vi "Laser manager 1.0BETA_withMotor.vi"() -> ()   [LabVIEW 2014]
uses:
  <vilib>/userdefined/High Color/IMAQdx.ctl
  Typedef/Consumer loop - States.ctl
  Typedef/UI data.ctl
  <vilib>/MakerHub/LINX/Public/Peripherals/Digital/Digital Write 1 Chan.vi
  <vilib>/MakerHub/LINX/Public/Peripherals/Digital/Digital Write N Chans.vi
  <vilib>/MakerHub/LINX/Private/Local IO/LinxDigitalWrite.vi
  <vilib>/MakerHub/LINX/Public/Utilities/Check Channel.vi
  <vilib>/MakerHub/LINX/Public/Utilities/Open Serial.vi
  <vilib>/MakerHub/LINX/Private/Utilties/Generate Error.vi
  <vilib>/vision/driver/NI_Vision_Acquisition_Software.lvlib
  <vilib>/MakerHub/LINX/LMH-LINX.lvlib
panel:
  in  "Move":bool
  in  "Absolute Y":dbl caption="Absolute Y [mm]"
  in  "Absolute X":dbl caption="Absolute X [mm]"
  in  "Delta Y":dbl caption="Delta Y [mm]"
  in  "Delta X":dbl caption="Delta X [mm]"
  in  "Move type":enum32{"Step mode", "\"Go to\" mode"}(radio)=enum."\"Go to\" mode"
  in  "Right":bool
  in  "Left":bool
  in  "Up":bool
  in  "Down":bool
  in  "Exit":bool
  out "Image":T1(plugin-control)
  in  "Tab Control":enum32{"Standard operations", "Refill", "Tools"}(tab)
  in  "Main - Open calib":bool
  in  "Go to calib":bool
  in  "Save calib":bool
  in  "Thyratron Bias [kV]":dbl=20.0
  in  "Test Laser":bool
  in  "Frequency [Hz]":u16=1 min=1 max=50 step=1
  in  "Beam Y":dbl=63.0 caption="Y" min=0.1 step=1.0 format="%#_gmm"
  in  "Beam X":dbl=1.0 caption="X" min=0.1 step=1.0 format="%#_gmm"
  in  "How to choose":bool
  in  "Load Pt2":bool
  out "X2":dbl format="%.2fmm"
  out "Y2":dbl format="%.2fmm"
  in  "Load Pt1":bool
  out "X1":dbl format="%.2fmm"
  out "Y1":dbl format="%.2fmm"
  in  "Abort":bool
  in  "Beam Overlap":dbl caption="Lateral Overlap [mm]" min=0.0 max=62.0 step=1.0
  in  "Shots/point":dbl=1.0 min=1.0 max=1000.0 step=1.0
  in  "Xspeed":dbl=1.0 caption="X speed [mm/s]" min=0.01 max=100.0 format="%#_3g"
  in  "Irradiate":bool
  out "Pressure":string caption="Pressure [mbar]"
  in  "Refill":bool
  in  "Purge Inert":bool
  in  "Purge Buffer":bool
  in  "Purge Rare":bool
  in  "Purge Halogen":bool
  in  "Set Gas Pressures [mbar]":T2={"Halogen"=80, "Rare"=60, "Buffer "=3160, "Inert"=0}
  out "Interface status":bool
  in  "Motor Enable":bool
  in  "Open GPIB interface":bool
  in  "Enable motors":bool
  in  "Find Origin":bool
  in  "Reset ESP":bool
  in  "Tools - Open Calib":bool
  in  "Open Attenuator":bool
  # "Free mode"
  # "LASER MANAGER 1.1 BETA"
  # "written by frax84"
  # "Energy Calibration"
  # "Laser Parameters"
  # "Beam parameters"
  # "Beam size"
  # "Motor path settings"
  # "Irradiation main controls"
  # "Purge Options"
  # "CAUTION\nEach purge operation \nlasts 5 seconds!"
  # "Reading is performed\nevery 5 seconds"
  # "Peripherals comunication"
  # "Gas mixing motor control"
  # "Motor Utilities"
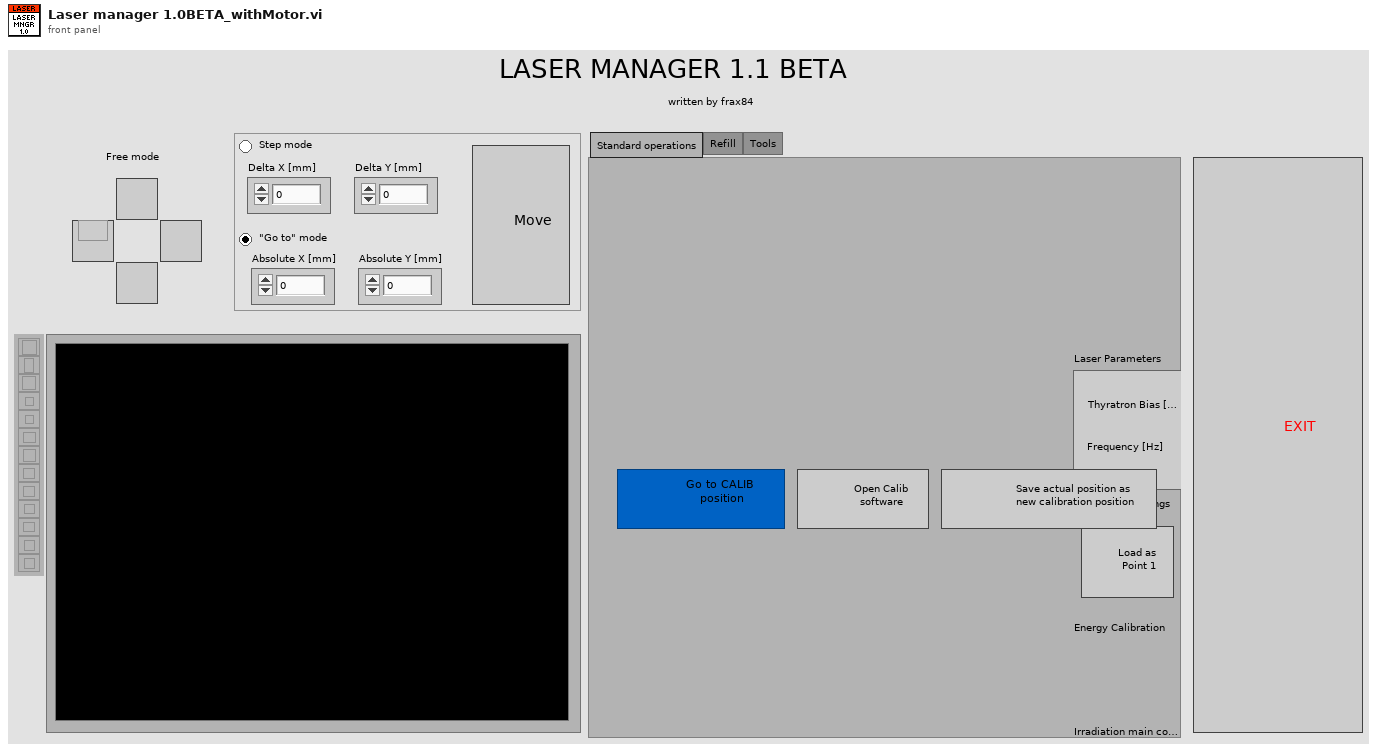
[diagram p1: front panel]
types:
  T1 = typedef "IMAQ Image.ctl" = refnum<image>
  T2 = cluster{"Halogen":u16, "Rare":u16, "Buffer ":u16, "Inert":u16}
  T3 = typedef "UI data.ctl" = cluster{"GPIB Addresses":cluster{"GPIB Motor":i16, "GPIB Laser":string}, "Beam size":cluster{"BeamX":dbl, "BeamY":dbl, "Beam Overlap":dbl}, "Motor speed":cluster{"Xspeed":dbl, " Yspeed":dbl}, "Laser parameters":cluster{"Thyratron Bias":dbl, "Frequency":u16, "Shots/Point":dbl}, "Irradiation points":cluster{"X1":dbl, "Y1":dbl, "X2":dbl, "Y2":dbl}, "Calibration Point":cluster{"Xcalib":dbl, "Ycalib":dbl}}
  T4 = typedef "Consumer loop - States.ctl" = enum16{"Idle", "Read Pressure", "Move up", "Move down", "Move left", "Move right", "Move to", "Move Delta", "Stop Motion", "Go to calib", "Check if move done", "Disable buttons", "Enable buttons", "Irradiation - Stop", "Irradiation - Check points", "Irradiation - Disable buttons", "Irradiation - Init position", "Irradiation - Check if done", "Irradiation - Sweep X", "Irradiation - Check X", "Irradiation - Check Y", "Irradiation - Sweep Y", "Irradiation - Enable buttons"}
  T5 = typedef "Image Type" = u32
  T6 = typedef "IMAQdx.ctl" = refnum<k21>
  T7 = enum8{"Enabled", "Disabled", "Disabled and Grayed Out"}
  T8 = typedef "LMH-LINX.lvlib/LINX Ref.ctl" = cluster{"IO":T9, "Interface":T10, "LINX Device Config":T11}
  T9 = typedef "LMH-LINX.lvlib/Platform.ctl" = enum16{"Remote", "Local"}
  T10 = typedef "LMH-LINX.lvlib/Interface.ctl" = enum16{"Serial", "TCP"}
  T11 = typedef "LMH-LINX.lvlib/Device.lvlib/LINX Device Config.ctl" = cluster{"Interface":T10, "COM Port":refnum<visa-resource-name>, "TCP Configuration":T12, "Device Family":u8, "Device ID":u8, "Device Name":string, "TCP Ref":refnum<k5>, "Channels":T13}
  T12 = typedef "LMH-LINX.lvlib/Device.lvlib/TCP Config.ctl" = cluster{"IP Address":string, "Port":u16}
  T13 = typedef "LMH-LINX.lvlib/Channels.ctl" = cluster{"DI":u8[], "DO":u8[], "AI":u8[], "AO":u8[], "PWM":u8[], "QE":u8[], "UART":u8[], "I2C 2":u8[], "SPI":u8[], "CAN":u8[], "Servo":u8[], "AI Ref (V)":dbl, "AI Resolution (Bits)":u8, "AO Ref (V)":dbl, "AO Resolution (Bits)":u8}
  T14 = cluster{"Global Rectangle":i32[], "Contours":cluster{"Contour Type":u32, "ROI Type":u32, "Points":i32[]}[]}
  T15 = cluster{"Global Rectangle[0]":i32, "Global Rectangle[1]":i32, "Global Rectangle[2]":i32, "Global Rectangle[3]":i32}
  T16 = cluster{"Consumer loop - States":T4, "Variant":variant}
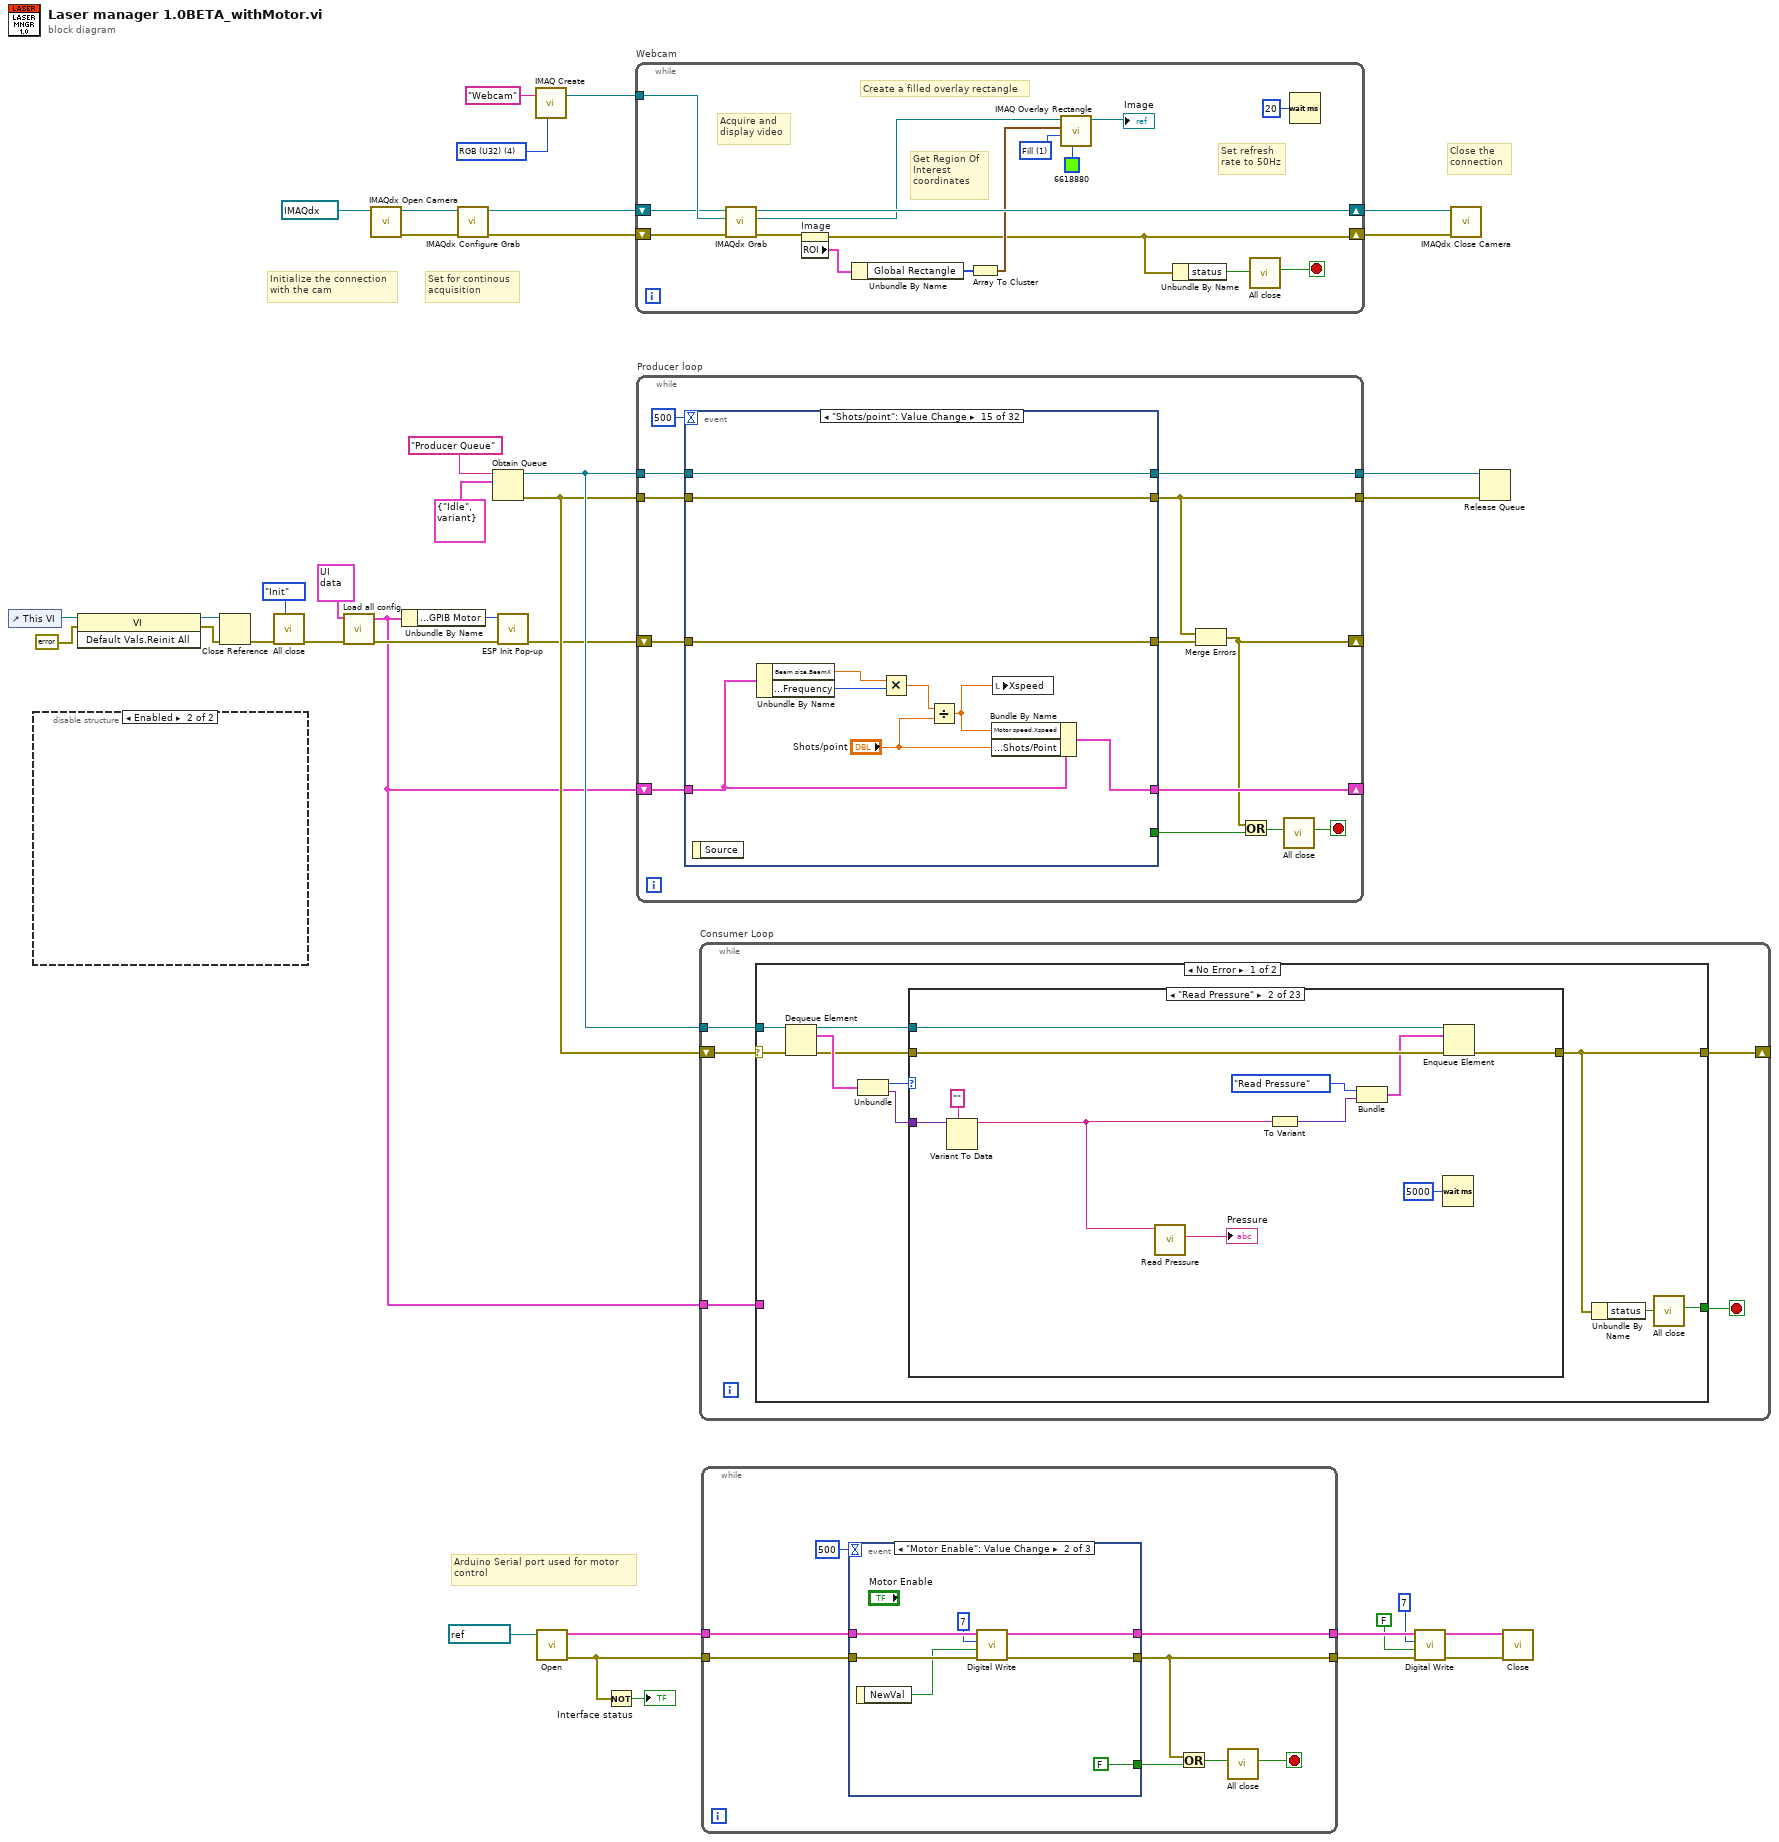
[diagram p0: block diagram]
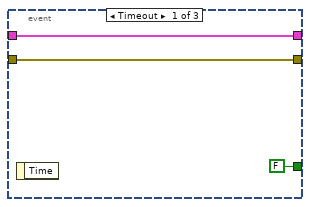
[diagram p2: hidden frame]
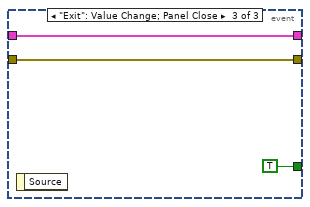
[diagram p3: hidden frame]
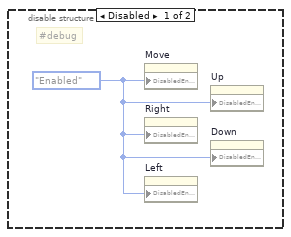
[diagram p4: hidden frame]
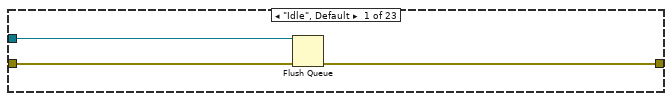
[diagram p5: hidden frame]
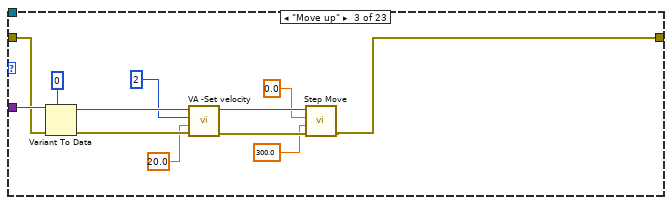
[diagram p6: hidden frame]
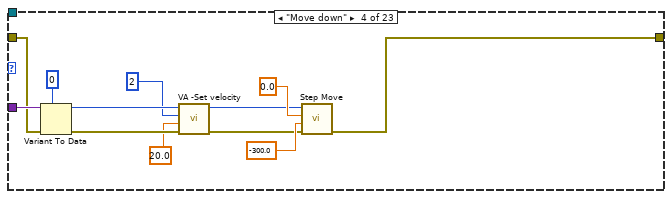
[diagram p7: hidden frame]
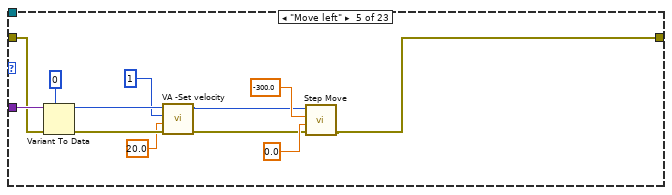
[diagram p8: hidden frame]
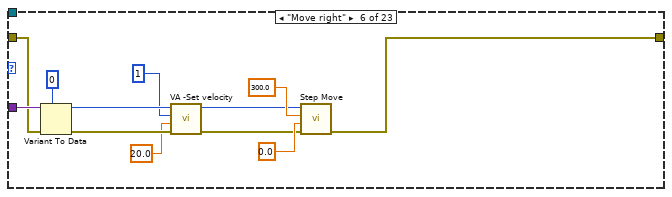
[diagram p9: hidden frame]
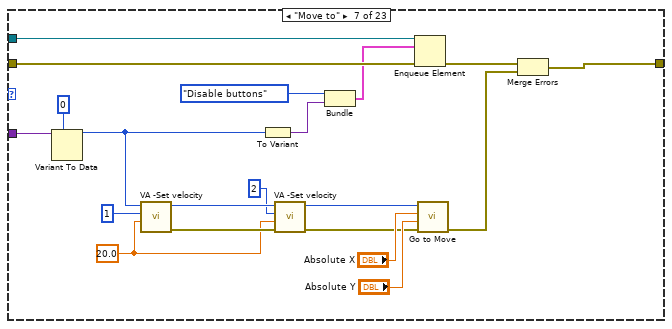
[diagram p10: hidden frame]
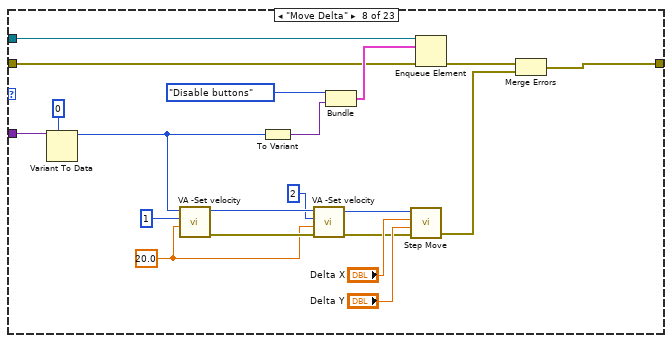
[diagram p11: hidden frame]
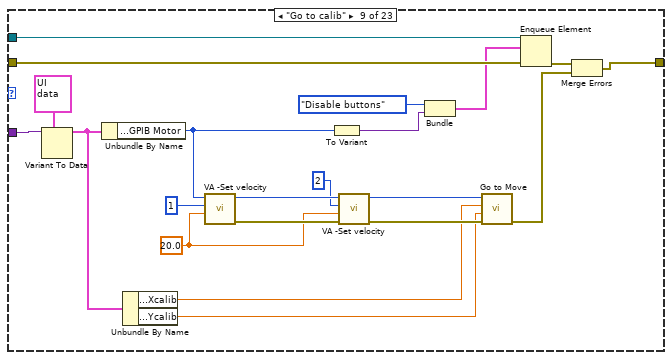
[diagram p12: hidden frame]
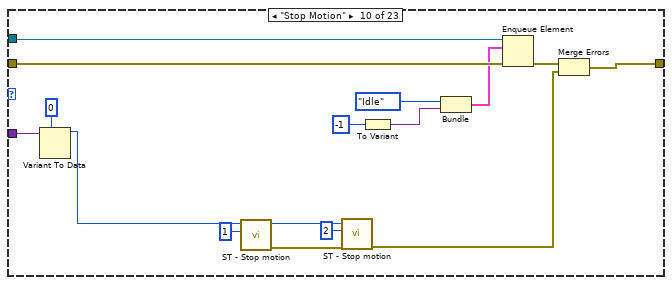
[diagram p13: hidden frame]
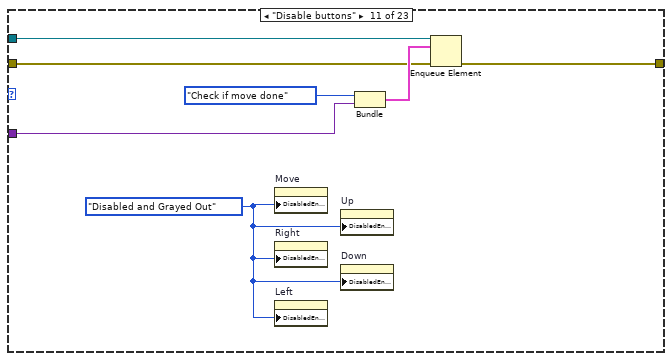
[diagram p14: hidden frame]
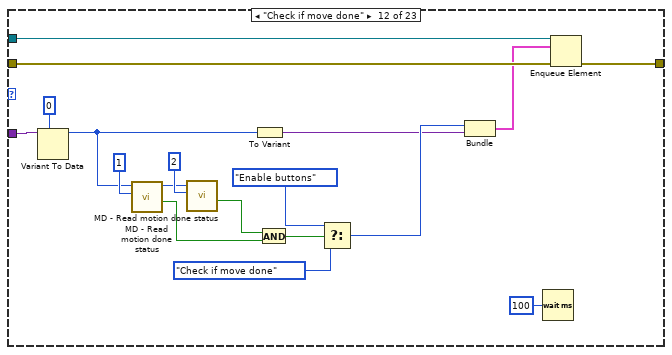
[diagram p15: hidden frame]
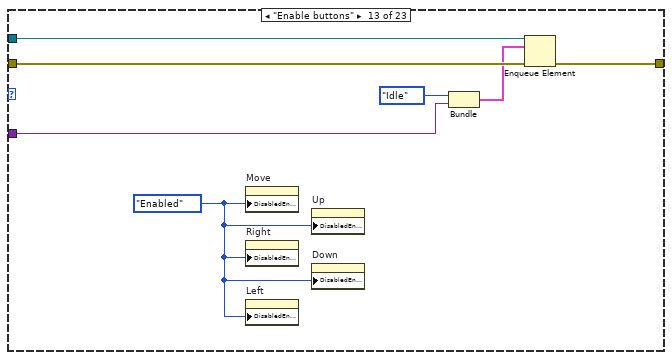
[diagram p16: hidden frame]
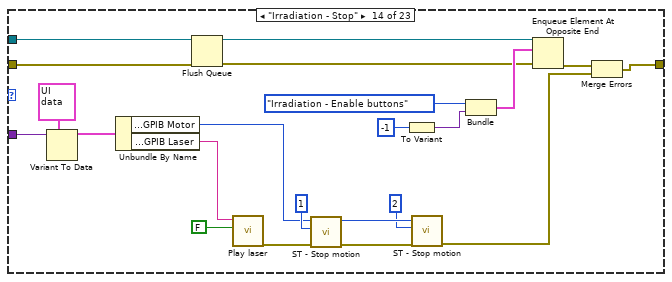
[diagram p17: hidden frame]
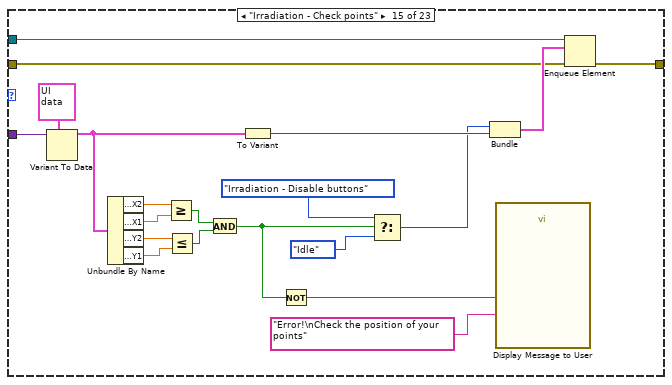
[diagram p18: hidden frame]
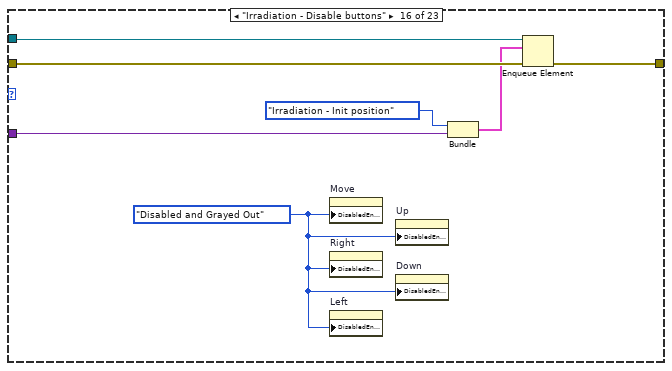
[diagram p19: hidden frame]
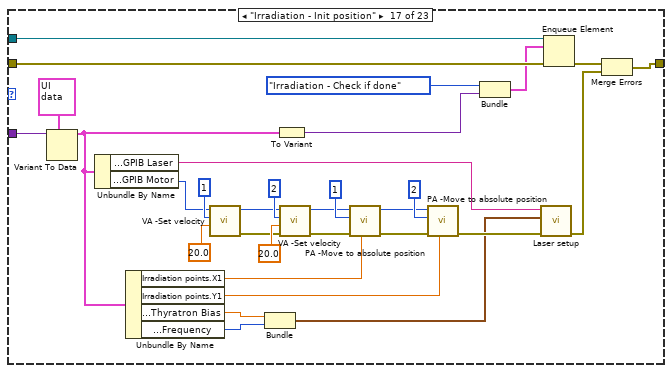
[diagram p20: hidden frame]
diagram:
  w32 = T5 4 items=["Grayscale (U8)", "Grayscale (I16)", "Grayscale (SGL)", "Complex (CSG)", "RGB (U32)", "HSL (U32)", "RGB (U64)", "Grayscale (U16)"] ("Image Type")
  # "Arduino Serial port used for motor\ncontrol"
  # "Close the \nconnection"
  # "Set for continous\nacquisition"
  # "Initialize the connection\nwith the cam"
  n1 = control-ref of="This VI"() -> (w15:refnum<vi>)
  n2 = disable-structure shown="Enabled" {
    frame Disabled {
      w39 = T7."Enabled" ("Disabled")
      # "#debug"
      n3 = property on="Move" class="Bool"("DisabledEnum"=w39) -> ()  [unwired: 2 in, 2 out]
      n4 = property on="Right" class="Bool (strict)"("DisabledEnum"=w39) -> ()  [unwired: 2 in, 2 out]
      n5 = property on="Left" class="Bool (strict)"("DisabledEnum"=w39) -> ()  [unwired: 2 in, 2 out]
      n6 = property on="Up" class="Bool (strict)"("DisabledEnum"=w39) -> ()  [unwired: 2 in, 2 out]
      n7 = property on="Down" class="Bool (strict)"("DisabledEnum"=w39) -> ()  [unwired: 2 in, 2 out]
    }
    frame Enabled {
    }
  }
  n8 = invoke class="VI" method="Default Vals.Reinit All"(reference=w15, error in=errorcluster {"status"=FALSE, "code"=0, "source"=""} ("Error In")) -> (reference out=w13:refnum<vi>, error out=w14:errorcluster)  [unwired: 1 in, 1 out]
  n9 = Close Reference(reference=w13, error in (no error)=w14) -> (error out=w12:errorcluster)
  n10 = call "All close.vi"("Operation (Check)"=enum16{"Init", "Check"}."Init" ("Operation"), "Error In"=w12) -> ("Error Out"=w18:errorcluster)  [unwired: 8 in, 1 out]
  n11 = call "Load all config.vi"("Error In"=w18, "UI data in"=T3 {"GPIB Addresses"={"GPIB Motor"=2, "GPIB Laser"="3"}, "Beam size"={"BeamX"=1.0, "BeamY"=63.0, "Beam Overlap"=0.0}, "Motor speed"={"Xspeed"=1.0, " Yspeed"=1.0}, "Laser parameters"={"Thyratron Bias"=20.0, "Frequency"=1, "Shots/Point"=1.0}, "Irradiation points"={"X1"=0.0, "Y1"=0.0, "X2"=0.0, "Y2"=0.0}, "Calibration Point"={"Xcalib"=0.0, "Ycalib"=0.0}} ("User Interface data")) -> ("Error Out"=w20:errorcluster, "UI data out"=w19:T3)  [unwired: 8 in]
  n12 = call <vilib>:"IMAQdx Open Camera.vi"("Session In"=T6 "cam1") -> ("error out"=w37:errorcluster, "Session Out"=w38:T6)  [unwired: 9 in]
  n13 = Unbundle By Name(w19) -> ("GPIB Addresses.GPIB Motor"=w23:i16)
  n14 = call <vilib>:"IMAQdx Configure Grab.vi"("error in"=w37, "Session In"=w38) -> ("error out"=w30:errorcluster, "Session Out"=w29:T6)  [unwired: 8 in]
  n15 = Obtain Queue(name (unnamed)="Producer Queue", element data type=cluster{"Consumer loop - States":T4, variant} {"Consumer loop - States"=enum."Idle", variant}) -> (queue out=w27:refnum<queue>, error out=w26:errorcluster)  [unwired: 3 in, 1 out]
  n16 = call "ESP Init Pop-up.vi"("Error In"=w20, "Address / Port in"=w23) -> ("Error Out"=w24:errorcluster)  [unwired: 9 in]
  n17 = call "IMAQ Create"("Image Name"="Webcam", "Image Type"=w32) -> ("New Image"=w33:T1)  [unwired: 3 in, 1 out]
  n18 = call-poly <vilib>:"Open.vi"("Serial Port"=refnum<visa-resource-name> "COM3" ("Arduino port:")) -> ("Error Out"=w7:errorcluster, "LINX Resource"=w10:T8)  [unwired: 8 in, 1 out]
  n19 = Not(x=w7) -> (.not. x?=→"Interface status":bool)
  n20 = while "Webcam" {
    shift-right: [w55] -> w35
    shift-left: w29 -> [w53]
    shift-right: [w41] -> w34
    shift-left: w30 -> [w52]
    tunnel: w33 -> [w54]
    stop <- w42 stop-if-true
    w45 = u32 1 items=["Frame", "Fill", "Highlight"] ("Drawing Mode (Frame)")
    # "Set refresh \nrate to 50Hz"
    # "Get Region Of \nInterest\ncoordinates"
    # "Create a filled overlay rectangle"
    # "Acquire and \ndisplay video"
    n21 = call <vilib>:"IMAQdx Grab.vi"("error in"=w52, "Image In"=w54, "Session In"=w53) -> ("error out"=w51:errorcluster, "Image Out"=w46:T1, "Session Out"=w55:T6)  [unwired: 5 in, 1 out]
    n22 = property on="Image" class="ImageControl"(error in=w51) -> (error out=w41:errorcluster, "ROI"=w50:T14)  [unwired: 1 in, 1 out]
    n23 = Unbundle By Name(w50) -> ("Global Rectangle"=w49:i32[])
    n24 = Array To Cluster(array=w49) -> (cluster=w48:T15)
    n25 = call "IMAQ Overlay Rectangle"("Color"=u32 6618880, "Drawing Mode (Frame)"=w45, "Rectangle"=w48, "Image"=w46) -> ("Image Out"=→"Image":T1)  [unwired: 6 in, 1 out]
    n26 = Unbundle By Name(w41) -> ("status"=w40:bool)
    n27 = call "All close.vi"("Close? (F)"=w40) -> ("Close"=w42:bool)  [unwired: 9 in, 1 out]
    n28 = Wait (ms)(milliseconds to wait=u32 20) -> ()  [unwired: 1 out]
  }
  n29 = while "Producer loop" {
    shift-right: [w59] -> _
    shift-left: w24 -> [w68]
    shift-right: [w66] -> _
    shift-left: w19 -> [w67]
    tunnel: w27 -> [w64]
    tunnel: w26 -> [w63]
    tunnel: [w58] -> w22
    tunnel: [w61] -> w21
    stop <- w56 stop-if-true
    n30 = event shown="[14] \"Shots/point\": Value Change" {
      selector: _ -> [_ _ _ _ _ _ _ _ _ _ _ _ _ _ _ _ _ _ _ _ _ _ _ _ _ _ _ _ _ _ _ _]
      dyn-events: _ -> [_ _ _ _ _ _ _ _ _ _ _ _ _ _ _ _ _ _ _ _ _ _ _ _ _ _ _ _ _ _ _ _]
      timeout: 500 -> [_ _ _ _ _ _ _ _ _ _ _ _ _ _ _ _ _ _ _ _ _ _ _ _ _ _ _ _ _ _ _ _]
      tunnel: w68 -> [w72 w87 w88 w101 w114 w127 w144 w163 w172 w185 w198 w208 w214 w235 w245 w255 w260 w270 w275 w284 w290 w297 w306 w315 w323 w331 w338 w346 w351 w375 w384 w390]
      tunnel: [w72 w87 w88 w101 w114 w127 w144 w151 w171 w184 w197 w207 w214 w235 w245 w255 w260 w270 w275 w283 w289 w296 w305 w314 w322 w330 w336 w347 w351 w375 w383 w394] -> w60
      tunnel: w67 -> [w71 w78 w93 w107 w118 w133 w141 w157 w169 w182 w192 w202 w210 w234 w241 w251 w263 w269 w278 w281 w287 w294 w304 w313 w321 w328 w337 w345 w355 w372 w382 w395]
      tunnel: [w71 w78 w93 w107 w118 w133 w141 w152 w166 w181 w192 w202 w210 w234 w239 w249 w261 w268 w276 w281 w287 w294 w304 w313 w321 w328 w337 w345 w355 w372 w382 w395] -> w66
      tunnel: [_ _ _ _ _ _ _ _ _ _ _ _ _ _ _ _ _ _ _ _ _ _ _ _ _ _ _ _ _ _ _ TRUE] -> w62
      tunnel: w64 -> [w70 w86 w97 w106 w120 w132 w148 w149 w165 w178 w191 w201 w221 w232 w238 w248 w259 w272 w274 w280 w286 w293 w299 w311 w319 w327 w335 w343 w363 w374 w379 w391]
      tunnel: w63 -> [w69 w85 w96 w105 w119 w131 w145 w150 w164 w177 w190 w200 w222 w233 w237 w247 w258 w271 w273 w279 w285 w292 w298 w310 w318 w326 w334 w342 w362 w373 w377 w392]
      tunnel: [w69 w73 w89 w102 w115 w128 w146 w150 w164 w177 w190 w200 w222 w233 w237 w247 w258 w271 w273 w279 w285 w292 w298 w310 w318 w326 w334 w342 w349 w368 w376 w392] -> w58
      tunnel: [w70 w74 w90 w103 w116 w129 w147 w149 w165 w178 w191 w201 w221 w232 w238 w248 w259 w272 w274 w280 w286 w293 w299 w311 w319 w327 w335 w343 w350 w369 w378 w391] -> w61
      event Timeout {
        # "Needed if error occurs"
        n31 = event-data() -> ()  [unwired: 1 in, 1 out]
      }
      event "Move": Value Change {
        n32 = event-data() -> ()  [unwired: 1 in, 1 out]
        n33 = Unbundle By Name(w78) -> ("GPIB Addresses.GPIB Motor"=w77:i16)
        n34 = Equal?(x="Move type", y=enum32{"Step mode", "\"Go to\" mode"}."\"Go to\" mode") -> (x = y?=w82:bool)
        n35 = To Variant(anything=w77) -> (Variant=w76:variant)
        n36 = Select(t=Consumer_loop_-_States."Move to" ("Consumer loop - States"), s=w82, f=Consumer_loop_-_States."Move Delta") -> (s? t:f=w81:T4)
        n37 = Bundle("f"=w81, "Variant"=w76) -> (w75:cluster{"f":T4, "Variant":variant})  [unwired: 1 in]
        n38 = Enqueue Element(queue=w86, element=w75, error in (no error)=w85) -> (queue out=w74:refnum<queue>, error out=w73:errorcluster)  [unwired: 1 in, 1 out]
      }
      event "Up": Value Change {
        n39 = event-data() -> ("NewVal"=w100:bool)  [unwired: 1 in]
        n40 = Unbundle By Name(w93) -> ("GPIB Addresses.GPIB Motor"=w91:i16)
        n41 = To Variant(anything=w91) -> (Variant=w92:variant)
        n42 = Select(t=Consumer_loop_-_States."Move up", s=w100, f=Consumer_loop_-_States."Stop Motion" ("Consumer loop - States")) -> (s? t:f=w95:T4)
        n43 = Bundle("Consumer loop - States"=w95, "Variant"=w92) -> (w94:T16)  [unwired: 1 in]
        n44 = Enqueue Element(queue=w97, element=w94, error in (no error)=w96) -> (queue out=w90:refnum<queue>, error out=w89:errorcluster)  [unwired: 1 in, 1 out]
      }
      event "Down": Value Change {
        n45 = event-data() -> ("NewVal"=w104:bool)  [unwired: 1 in]
        n46 = Unbundle By Name(w107) -> ("GPIB Addresses.GPIB Motor"=w108:i16)
        n47 = To Variant(anything=w108) -> (Variant=w109:variant)
        n48 = Select(t=Consumer_loop_-_States."Move down", s=w104, f=Consumer_loop_-_States."Stop Motion" ("Consumer loop - States")) -> (s? t:f=w111:T4)
        n49 = Bundle("Consumer loop - States"=w111, "Variant"=w109) -> (w110:T16)  [unwired: 1 in]
        n50 = Enqueue Element(queue=w106, element=w110, error in (no error)=w105) -> (queue out=w103:refnum<queue>, error out=w102:errorcluster)  [unwired: 1 in, 1 out]
      }
      event "Left": Value Change {
        n51 = event-data() -> ("NewVal"=w117:bool)  [unwired: 1 in]
        n52 = Unbundle By Name(w118) -> ("GPIB Addresses.GPIB Motor"=w126:i16)
        n53 = To Variant(anything=w126) -> (Variant=w125:variant)
        n54 = Select(t=Consumer_loop_-_States."Move left", s=w117, f=Consumer_loop_-_States."Stop Motion" ("Consumer loop - States")) -> (s? t:f=w123:T4)
        n55 = Bundle("Consumer loop - States"=w123, "Variant"=w125) -> (w124:T16)  [unwired: 1 in]
        n56 = Enqueue Element(queue=w120, element=w124, error in (no error)=w119) -> (queue out=w116:refnum<queue>, error out=w115:errorcluster)  [unwired: 1 in, 1 out]
      }
      event "Right": Value Change {
        n57 = event-data() -> ("NewVal"=w130:bool)  [unwired: 1 in]
        n58 = Unbundle By Name(w133) -> ("GPIB Addresses.GPIB Motor"=w139:i16)
        n59 = To Variant(anything=w139) -> (Variant=w138:variant)
        n60 = Select(t=Consumer_loop_-_States."Move right", s=w130, f=Consumer_loop_-_States."Stop Motion" ("Consumer loop - States")) -> (s? t:f=w136:T4)
        n61 = Bundle("Consumer loop - States"=w136, "Variant"=w138) -> (w137:T16)  [unwired: 1 in]
        n62 = Enqueue Element(queue=w132, element=w137, error in (no error)=w131) -> (queue out=w129:refnum<queue>, error out=w128:errorcluster)  [unwired: 1 in, 1 out]
      }
      event "Go to calib": Value Change {
        n63 = event-data() -> ()  [unwired: 1 in, 1 out]
        n64 = To Variant(anything=w141) -> (Variant=w140:variant)
        n65 = Bundle("Consumer loop - States"=Consumer_loop_-_States."Go to calib", "Variant"=w140) -> (w143:T16)  [unwired: 1 in]
        n66 = Enqueue Element(queue=w148, element=w143, error in (no error)=w145) -> (queue out=w147:refnum<queue>, error out=w146:errorcluster)  [unwired: 1 in, 1 out]
      }
      event "Save calib": Value Change {
        n67 = event-data() -> ()  [unwired: 1 in, 1 out]
        n68 = Unbundle By Name(w157) -> ("GPIB Addresses.GPIB Motor"=w162:i16)
        n69 = call "TP - Read actual position.vi"("error in"=w163, "Axis"=i8 1, "Address / Port"=w162) -> ("error out"=w160:errorcluster, "Query the current actual\nposition - read"=w156:dbl, "Address / Port dup"=w159:i16)  [unwired: 5 in, 1 out]
        n70 = call "TP - Read actual position.vi"("error in"=w160, "Axis"=i8 2, "Address / Port"=w159) -> ("error out"=w154:errorcluster, "Query the current actual\nposition - read"=w155:dbl)  [unwired: 5 in, 2 out]
        n71 = Bundle By Name(cluster=w157, "Calibration Point.Ycalib"=w155, "Calibration Point.Xcalib"=w156) -> (w153:T3)
        n72 = call "Save calib config.vi"("Error In"=w154, "UI data in"=w153) -> ("Error Out"=w151:errorcluster, "UI data out"=w152:T3)  [unwired: 8 in]
      }
      event "Load Pt1": Value Change {
        n73 = event-data() -> ()  [unwired: 1 in, 1 out]
        n74 = Unbundle By Name(w169) -> ("GPIB Addresses.GPIB Motor"=w170:i16)
        n75 = call "TP - Read actual position.vi"("error in"=w172, "Axis"=i8 1, "Address / Port"=w170) -> ("error out"=w175:errorcluster, "Query the current actual\nposition - read"=w168:dbl, "Address / Port dup"=w176:i16)  [unwired: 5 in, 1 out]
        "X1" <- w168
        n76 = call "TP - Read actual position.vi"("error in"=w175, "Axis"=i8 2, "Address / Port"=w176) -> ("error out"=w171:errorcluster, "Query the current actual\nposition - read"=w167:dbl)  [unwired: 5 in, 2 out]
        "Y1" <- w167
        n77 = Bundle By Name(cluster=w169, "Irradiation points.Y1"=w167, "Irradiation points.X1"=w168) -> (w166:T3)
      }
      event "Load Pt2": Value Change {
        n78 = event-data() -> ()  [unwired: 1 in, 1 out]
        n79 = Unbundle By Name(w182) -> ("GPIB Addresses.GPIB Motor"=w183:i16)
        n80 = call "TP - Read actual position.vi"("error in"=w185, "Axis"=i8 1, "Address / Port"=w183) -> ("error out"=w188:errorcluster, "Query the current actual\nposition - read"=w180:dbl, "Address / Port dup"=w189:i16)  [unwired: 5 in, 1 out]
        "X2" <- w180
        n81 = call "TP - Read actual position.vi"("error in"=w188, "Axis"=i8 2, "Address / Port"=w189) -> ("error out"=w184:errorcluster, "Query the current actual\nposition - read"=w179:dbl)  [unwired: 5 in, 2 out]
        "Y2" <- w179
        n82 = Bundle By Name(cluster=w182, "Irradiation points.Y2"=w179, "Irradiation points.X2"=w180) -> (w181:T3)
      }
      event "Tools - Open Calib", "Main - Open calib": Value Change {
        n83 = event-data() -> ()  [unwired: 1 in, 1 out]
        n84 = call <vilib>:"Application Directory.vi"() -> ("Application Directory"=w196:path)
        n85 = Build Path(base path=w196, name or relative path="External software\\Thorlabs\\Optical Power Meter Utility.exe" ("command line")) -> (appended path=w195:path)
        n86 = Path To String(path=w195) -> (string=w193:string)
        n87 = call <vilib>:"System Exec.vi"("wait until completion? (T)"=FALSE, "error in (no error)"=w198, "command line"=w193) -> ("error out"=w197:errorcluster)  [unwired: 5 in, 3 out]
      }
      event "Open Attenuator": Value Change {
        n88 = event-data() -> ()  [unwired: 1 in, 1 out]
        n89 = call <vilib>:"Application Directory.vi"() -> ("Application Directory"=w206:path)
        n90 = Build Path(base path=w206, name or relative path="External software\\Coherent\\CohrAttenuatorApp.exe" ("command line")) -> (appended path=w205:path)
        n91 = Path To String(path=w205) -> (string=w203:string)
        n92 = call <vilib>:"System Exec.vi"("wait until completion? (T)"=FALSE, "error in (no error)"=w208, "command line"=w203) -> ("error out"=w207:errorcluster)  [unwired: 5 in, 3 out]
      }
      event "Open GPIB interface": Value Change {
        n93 = event-data() -> ()  [unwired: 1 in, 1 out]
        n94 = call <vilib>:"Application Directory.vi"() -> ("Application Directory"=w213:path)
        n95 = Build Path(base path=w213, name or relative path="Utilities\\GPIB \nSimple Interface.vi") -> (appended path=w211:path)
        n96 = Open VI Reference(vi path=w211) -> (vi reference=w219:refnum<vi>, error out=w216:errorcluster)  [unwired: 5 in]
        n97 = property class="VI"(reference=w219, error in=w216, "Front Panel Window:Open"=TRUE) -> (reference out=w218:refnum<vi>, error out=w215:errorcluster)
        n98 = invoke class="VI" method="Run VI"(reference=w218, error in=w215, "Wait until done"=FALSE) -> ()  [unwired: 2 in, 5 out]
      }
      event "How to choose": Value Change {
        n99 = event-data() -> ()  [unwired: 1 in, 1 out]
        n100 = call <vilib>:"Application Directory.vi"() -> ("Application Directory"=w225:path)
        n101 = Build Path(base path=w225, name or relative path="SubVIs\\How to.vi") -> (appended path=w223:path)
        n102 = Open VI Reference(vi path=w223) -> (vi reference=w230:refnum<vi>, error out=w227:errorcluster)  [unwired: 5 in]
        n103 = property class="VI"(reference=w230, error in=w227, "Front Panel Window:Open"=TRUE) -> (reference out=w229:refnum<vi>, error out=w226:errorcluster)
        n104 = invoke class="VI" method="Run VI"(reference=w229, error in=w226, "Wait until done"=FALSE) -> ()  [unwired: 2 in, 5 out]
      }
      event "Shots/point": Value Change {
        n105 = event-data() -> ()  [unwired: 1 in, 1 out]
        n106 = Unbundle By Name(w241) -> ("Beam size.BeamX"=w244:dbl, "Laser parameters.Frequency"=w243:u16)
        n107 = Multiply(x=w244, y=w243) -> (x*y=w242:dbl)
        n108 = Divide(x=w242, y="Shots/point") -> (x/y=w236:dbl)
        n109 = Bundle By Name(cluster=w241, "Motor speed.Xspeed"=w236, "Laser parameters.Shots/Point"="Shots/point") -> (w239:T3)
        n110 = local write "Xspeed"(w236) -> ()
      }
      event "Xspeed": Value Change {
        n111 = event-data() -> ()  [unwired: 1 in, 1 out]
        n112 = Unbundle By Name(w251) -> ("Beam size.BeamX"=w254:dbl, "Laser parameters.Frequency"=w253:u16)
        n113 = Multiply(x=w254, y=w253) -> (x*y=w252:dbl)
        n114 = Divide(x=w252, y="Xspeed") -> (x/y=w246:dbl)
        n115 = local write "Shots/point"(w246) -> ()
        n116 = Bundle By Name(cluster=w251, "Laser parameters.Shots/Point"=w246, "Motor speed.Xspeed"="Xspeed") -> (w249:T3)
      }
      event "Frequency [Hz]", "Beam X": Value Change {
        n117 = event-data() -> ()  [unwired: 1 in, 1 out]
        n118 = Unbundle By Name(w263) -> ("Laser parameters.Shots/Point"=w264:dbl)
        n119 = Multiply(x="Frequency [Hz]", y="Beam X") -> (x*y=w265:dbl)
        n120 = Divide(x=w265, y=w264) -> (x/y=w257:dbl)
        n121 = local write "Xspeed"(w257) -> ()
        n122 = Bundle By Name(cluster=w263, "Laser parameters.Frequency"="Frequency [Hz]", "Beam size.BeamX"="Beam X", "Motor speed.Xspeed"=w257) -> (w261:T3)
      }
      event "Beam Overlap", "Beam Y": Value Change {
        n123 = event-data() -> ()  [unwired: 1 in, 1 out]
        n124 = Bundle By Name(cluster=w269, "Beam size.BeamY"="Beam Y", "Beam size.Beam Overlap"="Beam Overlap") -> (w268:T3)
      }
      event "Thyratron Bias [kV]": Value Change {
        n125 = event-data() -> ()  [unwired: 1 in, 1 out]
        n126 = Bundle By Name(cluster=w278, "Laser parameters.Thyratron Bias"="Thyratron Bias [kV]") -> (w276:T3)
      }
      event "Find Origin": Value Change {
        n127 = event-data() -> ()  [unwired: 1 in, 1 out]
        n128 = Unbundle By Name(w281) -> ("GPIB Addresses.GPIB Motor"=w282:i16)
        n129 = call "Find Origin.vi"("Error In"=w284, "Address / Port"=w282) -> ("Error Out"=w283:errorcluster)  [unwired: 8 in, 1 out]
      }
      event "Enable motors": Value Change {
        n130 = event-data() -> ()  [unwired: 1 in, 1 out]
        n131 = Unbundle By Name(w287) -> ("GPIB Addresses.GPIB Motor"=w288:i16)
        n132 = call "Enable Motor.vi"("Error In"=w290, "On/Off"=enum16{"On", "Off"}."On", "Address / Port"=w288) -> ("Error Out"=w289:errorcluster)  [unwired: 7 in, 1 out]
      }
      event "Reset ESP": Value Change {
        n133 = event-data() -> ()  [unwired: 1 in, 1 out]
        n134 = Unbundle By Name(w294) -> ("GPIB Addresses.GPIB Motor"=w295:i16)
        n135 = call "RS - Reset the controller.vi"("error in"=w297, "Address / Port"=w295) -> ("error out"=w296:errorcluster)  [unwired: 6 in, 1 out]
      }
      event "Test Laser": Value Change {
        n136 = event-data() -> ("NewVal"=w307:bool)  [unwired: 1 in]
        n137 = Unbundle By Name(w304) -> ("GPIB Addresses.GPIB Laser"=w303:string, "Laser parameters.Thyratron Bias"=w302:dbl, "Laser parameters.Frequency"=w301:u16)
        n138 = Bundle("Thyratron Bias"=w302, "Frequency"=w301) -> (w300:cluster{"Thyratron Bias":dbl, "Frequency":u16})  [unwired: 1 in]
        n139 = call "Laser setup.vi"("Error In"=w306, "Laser Parameters"=w300, "GPIB Address"=w303) -> ("Error Out"=w308:errorcluster, "GPIB Address out"=w309:string)  [unwired: 7 in]
        n140 = call "Play laser.vi"("Error In"=w308, "Laser On"=w307, "GPIB Address"=w309) -> ("Error Out"=w305:errorcluster)  [unwired: 7 in, 1 out]
      }
      event "Purge Halogen": Value Change {
        n141 = event-data() -> ()  [unwired: 1 in, 1 out]
        n142 = Unbundle By Name(w313) -> ("GPIB Addresses.GPIB Laser"=w312:string)
        n143 = call "Purge Line.vi"("Error In"=w315, "Gas"=enum16{"Halogen", "Rare", "Buffer", "Inert"}."Halogen", "GPIB Address"=w312) -> ("Error Out"=w314:errorcluster)  [unwired: 7 in, 1 out]
        n144 = Wait (ms)(milliseconds to wait=u32 6000) -> ()  [unwired: 1 out]
      }
      event "Purge Rare": Value Change {
        n145 = event-data() -> ()  [unwired: 1 in, 1 out]
        n146 = Unbundle By Name(w321) -> ("GPIB Addresses.GPIB Laser"=w320:string)
        n147 = call "Purge Line.vi"("Error In"=w323, "Gas"=enum16{"Halogen", "Rare", "Buffer", "Inert"}."Rare", "GPIB Address"=w320) -> ("Error Out"=w322:errorcluster)  [unwired: 7 in, 1 out]
        n148 = Wait (ms)(milliseconds to wait=u32 6000) -> ()  [unwired: 1 out]
      }
      event "Purge Buffer": Value Change {
        n149 = event-data() -> ()  [unwired: 1 in, 1 out]
        n150 = Unbundle By Name(w328) -> ("GPIB Addresses.GPIB Laser"=w329:string)
        n151 = call "Purge Line.vi"("Error In"=w331, "Gas"=enum16{"Halogen", "Rare", "Buffer", "Inert"}."Buffer", "GPIB Address"=w329) -> ("Error Out"=w330:errorcluster)  [unwired: 7 in, 1 out]
        n152 = Wait (ms)(milliseconds to wait=u32 6000) -> ()  [unwired: 1 out]
      }
      event "Purge Inert": Value Change {
        n153 = event-data() -> ()  [unwired: 1 in, 1 out]
        n154 = Unbundle By Name(w337) -> ("GPIB Addresses.GPIB Laser"=w339:string)
        n155 = call "Purge Line.vi"("Error In"=w338, "Gas"=enum16{"Halogen", "Rare", "Buffer", "Inert"}."Inert", "GPIB Address"=w339) -> ("Error Out"=w336:errorcluster)  [unwired: 7 in, 1 out]
        n156 = Wait (ms)(milliseconds to wait=u32 6000) -> ()  [unwired: 1 out]
      }
      event "Refill": Value Change {
        n157 = event-data() -> ()  [unwired: 1 in, 1 out]
        n158 = Unbundle By Name(w345) -> ("GPIB Addresses.GPIB Laser"=w344:string)
        n159 = call "New Fill.vi"("Error In"=w346, "Gas settings"="Set Gas Pressures [mbar]", "GPIB Address"=w344) -> ("Error Out"=w347:errorcluster)  [unwired: 7 in, 1 out]
      }
      event "Tab Control": Value Change {
        # "If the Refill tab is chosen pressure is read every 5 seconds"
        n160 = event-data() -> ()  [unwired: 1 in, 1 out]
        n161 = Unbundle By Name(w355) -> ("GPIB Addresses.GPIB Laser"=w354:string)
        n162 = Equal?(x="Tab Control", y=enum32{"Standard operations", "Refill", "Tools"}."Refill") -> (x = y?=w359:bool)
        n163 = To Variant(anything=w354) -> (Variant=w353:variant)
        n164 = Select(t=Consumer_loop_-_States."Read Pressure" ("Consumer loop - States"), s=w359, f=Consumer_loop_-_States."Idle") -> (s? t:f=w356:T4)
        n165 = Bundle("f"=w356, "Variant"=w353) -> (w352:cluster{"f":T4, "Variant":variant})  [unwired: 1 in]
        n166 = Enqueue Element(queue=w363, element=w352, error in (no error)=w362) -> (queue out=w350:refnum<queue>, error out=w349:errorcluster)  [unwired: 1 in, 1 out]
      }
      event "Irradiate": Value Change {
        n167 = event-data() -> ("NewVal"=w367:bool)  [unwired: 1 in]
        n168 = To Variant(anything=w372) -> (Variant=w371:variant)
        n169 = Select(t=Consumer_loop_-_States."Irradiation - Check points" ("Consumer loop - States"), s=w367, f=Consumer_loop_-_States."Irradiation - Stop") -> (s? t:f=w365:T4)
        n170 = Bundle("f"=w365, "Variant"=w371) -> (w370:cluster{"f":T4, "Variant":variant})  [unwired: 1 in]
        n171 = Enqueue Element(queue=w374, element=w370, error in (no error)=w373) -> (queue out=w369:refnum<queue>, error out=w368:errorcluster)  [unwired: 1 in, 1 out]
      }
      event "Abort": Value Change {
        n172 = event-data() -> ()  [unwired: 1 in, 1 out]
        n173 = Unbundle By Name(w382) -> ("GPIB Addresses.GPIB Motor"=w381:i16, "GPIB Addresses.GPIB Laser"=w380:string)
        n174 = Flush Queue(queue=w379, error in (no error)=w377) -> (queue out=w378:refnum<queue>, error out=w376:errorcluster)  [unwired: 1 out]
        n175 = call "AB - Abort Motion.vi"("error in"=w384, "Address / Port"=w381) -> ("error out"=w386:errorcluster)  [unwired: 9 in]
        n176 = call "Play laser.vi"("Error In"=w386, "Laser On"=FALSE, "GPIB Address"=w380) -> ("Error Out"=w383:errorcluster)  [unwired: 7 in, 1 out]
      }
      event "Exit": Value Change {
        n177 = event-data() -> ()  [unwired: 1 in, 1 out]
        n178 = Unbundle By Name(w395) -> ("GPIB Addresses.GPIB Motor"=w388:i16, "GPIB Addresses.GPIB Laser"=w393:string)
        n179 = call "ST - Stop motion.vi"("error in"=w390, "Axis"=i8 1, "Address / Port"=w388) -> ("error out"=w389:errorcluster)  [unwired: 6 in, 2 out]
        n180 = call "Play laser.vi"("Error In"=w389, "Laser On"=FALSE, "GPIB Address"=w393) -> ("Error Out"=w394:errorcluster)  [unwired: 7 in, 1 out]
      }
    }
    n181 = Merge Errors(w58, w60) -> (w59:errorcluster)
    n182 = Or(x=w59, y=w62) -> (x .or. y?=w57:bool)
    n183 = call "All close.vi"("Close? (F)"=w57) -> ("Close"=w56:bool)  [unwired: 9 in, 1 out]
  }
  n184 = while "Consumer Loop" {
    tunnel: w27 -> [w402]
    shift-right: [w401] -> _
    shift-left: w26 -> [w400]
    tunnel: w19 -> [w398]
    stop <- w399 stop-if-true
    n185 = case shown="No Error" w400 {
      selector: w400 -> [w406 w788]
      tunnel: w402 -> [w412 _]
      tunnel: [w404 w785] -> w401
      tunnel: [w405 TRUE] -> w399
      tunnel: w398 -> [_ w791]
      frame No Error {
        n186 = Dequeue Element(queue=w412, error in (no error)=w406) -> (queue out=w408:refnum<queue>, element=w411:cluster{"Consumer loop - States":T4, variant}, error out=w409:errorcluster)  [unwired: 1 in, 1 out]
        n187 = Unbundle(w411) -> ("Consumer loop - States"=w410:T4, w407:variant)
        n188 = case shown="\"Read Pressure\"" w410 {
          tunnel: w409 -> [w414 w424 w436 w448 w460 w472 w489 w507 w522 w551 w554 w568 w582 w585 w621 w630 w640 w682 w698 w717 w743 w772 w780]
          tunnel: w408 -> [w415 w425 _ _ _ _ w490 w508 w523 w550 w555 w569 w583 w595 w622 w631 w641 w683 w699 w716 w742 w773 w779]
          tunnel: w407 -> [_ w420 w438 w449 w461 w473 w492 w512 w535 w549 w553 w575 w578 w599 w625 w626 w650 w685 w701 w724 w748 w774 w777]
          tunnel: [w413 w416 w429 w439 w452 w465 w484 w504 w516 w541 w552 w559 w577 w598 w612 w629 w633 w667 w691 w710 w736 w770 w778] -> w404
          frame "Idle", Default {
            n189 = Flush Queue(queue=w415, error in (no error)=w414) -> (error out=w413:errorcluster)  [unwired: 2 out]
          }
          frame "Read Pressure" {
            n190 = Variant To Data(type="" ("Instrument GPIB Addresses.GPIB Laser"), Variant=w420) -> (data=w417:string)  [unwired: 1 in, 1 out]
            n191 = call "Read Pressure.vi"("GPIB Address"=w417) -> ("Pressure [mbar]"=→"Pressure":string)  [unwired: 8 in, 2 out]
            n192 = To Variant(anything=w417) -> (Variant=w422:variant)
            n193 = Bundle("Consumer loop - States"=Consumer_loop_-_States."Read Pressure", "Variant"=w422) -> (w421:T16)  [unwired: 1 in]
            n194 = Wait (ms)(milliseconds to wait=u32 5000) -> ()  [unwired: 1 out]
            n195 = Enqueue Element(queue=w425, element=w421, error in (no error)=w424) -> (error out=w416:errorcluster)  [unwired: 1 in, 2 out]
          }
          frame "Move up" {
            n196 = Variant To Data(error in=w436, type=i16 0 ("Address / Port"), Variant=w438) -> (data=w434:i16, error out=w435:errorcluster)
            n197 = call "VA -Set velocity.vi"("error in"=w435, "Velocity\nset"=20.0 ("Velocity\nset"), "Axis #"=i8 2, "Address / Port"=w434) -> ("error out"=w431:errorcluster, "Address / Port dup"=w430:i16)  [unwired: 4 in, 2 out]
            n198 = call "Step Move.vi"("Error In"=w431, "Delta Y"=300.0 ("Move to travel limit\nset (+ or - )"), "Delta X"=0.0, "Address/Port in"=w430) -> ("Error Out"=w429:errorcluster)  [unwired: 6 in, 1 out]
          }
          frame "Move down" {
            n199 = Variant To Data(error in=w448, type=i16 0 ("Address / Port"), Variant=w449) -> (data=w447:i16, error out=w446:errorcluster)
            n200 = call "VA -Set velocity.vi"("error in"=w446, "Velocity\nset"=20.0 ("Velocity\nset"), "Axis #"=i8 2, "Address / Port"=w447) -> ("error out"=w440:errorcluster, "Address / Port dup"=w441:i16)  [unwired: 4 in, 2 out]
            n201 = call "Step Move.vi"("Error In"=w440, "Delta Y"=-300.0 ("Move to travel limit\nset (+ or - )"), "Delta X"=0.0, "Address/Port in"=w441) -> ("Error Out"=w439:errorcluster)  [unwired: 6 in, 1 out]
          }
          frame "Move left" {
            n202 = Variant To Data(error in=w460, type=i16 0 ("Address / Port"), Variant=w461) -> (data=w458:i16, error out=w459:errorcluster)
            n203 = call "VA -Set velocity.vi"("error in"=w459, "Velocity\nset"=20.0 ("Velocity\nset"), "Axis #"=i8 1, "Address / Port"=w458) -> ("error out"=w451:errorcluster, "Address / Port dup"=w453:i16)  [unwired: 4 in, 2 out]
            n204 = call "Step Move.vi"("Error In"=w451, "Delta Y"=0.0 ("Move to travel limit\nset (+ or - )"), "Delta X"=-300.0, "Address/Port in"=w453) -> ("Error Out"=w452:errorcluster)  [unwired: 6 in, 1 out]
          }
          frame "Move right" {
            n205 = Variant To Data(error in=w472, type=i16 0 ("Address / Port"), Variant=w473) -> (data=w470:i16, error out=w471:errorcluster)
            n206 = call "VA -Set velocity.vi"("error in"=w471, "Velocity\nset"=20.0 ("Velocity\nset"), "Axis #"=i8 1, "Address / Port"=w470) -> ("error out"=w463:errorcluster, "Address / Port dup"=w464:i16)  [unwired: 4 in, 2 out]
            n207 = call "Step Move.vi"("Error In"=w463, "Delta Y"=0.0 ("Move to travel limit\nset (+ or - )"), "Delta X"=300.0, "Address/Port in"=w464) -> ("Error Out"=w465:errorcluster)  [unwired: 6 in, 1 out]
          }
          frame "Move to" {
            w477 = 20.0 ("Velocity\nset")
            n208 = Variant To Data(type=i16 0 ("Instrument GPIB Addresses.GPIB Motor"), Variant=w492) -> (data=w478:i16)  [unwired: 1 in, 1 out]
            n209 = call "VA -Set velocity.vi"("Velocity\nset"=w477, "Axis #"=i8 1, "Address / Port"=w478) -> ("error out"=w479:errorcluster, "Address / Port dup"=w480:i16)  [unwired: 5 in, 2 out]
            n210 = To Variant(anything=w478) -> (Variant=w486:variant)
            n211 = call "VA -Set velocity.vi"("error in"=w479, "Velocity\nset"=w477, "Axis #"=i8 2, "Address / Port"=w480) -> ("error out"=w482:errorcluster, "Address / Port dup"=w481:i16)  [unwired: 4 in, 2 out]
            n212 = Bundle("Consumer loop - States"=Consumer_loop_-_States."Disable buttons", "Variant"=w486) -> (w487:T16)  [unwired: 1 in]
            n213 = Enqueue Element(queue=w490, element=w487, error in (no error)=w489) -> (error out=w485:errorcluster)  [unwired: 1 in, 2 out]
            n214 = call "Go to Move.vi"("Error In"=w482, "Absolute Y"="Absolute Y", "Absolute X"="Absolute X", "Address/Port in"=w481) -> ("Error Out"=w483:errorcluster)  [unwired: 6 in, 1 out]
            n215 = Merge Errors(w485, w483) -> (w484:errorcluster)
          }
          frame "Move Delta" {
            w500 = 20.0 ("Velocity\nset")
            n216 = Variant To Data(type=i16 0 ("Instrument GPIB Addresses.GPIB Motor"), Variant=w512) -> (data=w495:i16)  [unwired: 1 in, 1 out]
            n217 = call "VA -Set velocity.vi"("Velocity\nset"=w500, "Axis #"=i8 1, "Address / Port"=w495) -> ("error out"=w501:errorcluster, "Address / Port dup"=w502:i16)  [unwired: 5 in, 2 out]
            n218 = To Variant(anything=w495) -> (Variant=w506:variant)
            n219 = call "VA -Set velocity.vi"("error in"=w501, "Velocity\nset"=w500, "Axis #"=i8 2, "Address / Port"=w502) -> ("error out"=w497:errorcluster, "Address / Port dup"=w496:i16)  [unwired: 4 in, 2 out]
            n220 = Bundle("Consumer loop - States"=Consumer_loop_-_States."Disable buttons", "Variant"=w506) -> (w509:T16)  [unwired: 1 in]
            n221 = call "Step Move.vi"("Error In"=w497, "Delta Y"="Delta Y", "Delta X"="Delta X", "Address/Port in"=w496) -> ("Error Out"=w503:errorcluster)  [unwired: 6 in, 1 out]
            n222 = Enqueue Element(queue=w508, element=w509, error in (no error)=w507) -> (error out=w505:errorcluster)  [unwired: 1 in, 2 out]
            n223 = Merge Errors(w505, w503) -> (w504:errorcluster)
          }
          frame "Go to calib" {
            w527 = 20.0 ("Velocity\nset")
            n224 = Variant To Data(type=T3 {"GPIB Addresses"={"GPIB Motor"=2, "GPIB Laser"="3"}, "Beam size"={"BeamX"=0.0, "BeamY"=0.0, "Beam Overlap"=0.0}, "Motor speed"={"Xspeed"=0.0, " Yspeed"=0.0}, "Laser parameters"={"Thyratron Bias"=20.0, "Frequency"=0, "Shots/Point"=0.0}, "Irradiation points"={"X1"=0.0, "Y1"=0.0, "X2"=0.0, "Y2"=0.0}, "Calibration Point"={"Xcalib"=0.0, "Ycalib"=0.0}} ("User Interface data"), Variant=w535) -> (data=w526:T3)  [unwired: 1 in, 1 out]
            n225 = Unbundle By Name(w526) -> ("GPIB Addresses.GPIB Motor"=w520:i16)
            n226 = Unbundle By Name(w526) -> ("Calibration Point.Xcalib"=w525:dbl, "Calibration Point.Ycalib"=w524:dbl)
            n227 = call "VA -Set velocity.vi"("Velocity\nset"=w527, "Axis #"=i8 1, "Address / Port"=w520) -> ("error out"=w530:errorcluster, "Address / Port dup"=w531:i16)  [unwired: 5 in, 2 out]
            n228 = To Variant(anything=w520) -> (Variant=w519:variant)
            n229 = call "VA -Set velocity.vi"("error in"=w530, "Velocity\nset"=w527, "Axis #"=i8 2, "Address / Port"=w531) -> ("error out"=w533:errorcluster, "Address / Port dup"=w532:i16)  [unwired: 4 in, 2 out]
            n230 = Bundle("Consumer loop - States"=Consumer_loop_-_States."Disable buttons", "Variant"=w519) -> (w518:T16)  [unwired: 1 in]
            n231 = call "Go to Move.vi"("Error In"=w533, "Absolute Y"=w524, "Absolute X"=w525, "Address/Port in"=w532) -> ("Error Out"=w515:errorcluster)  [unwired: 6 in, 1 out]
            n232 = Enqueue Element(queue=w523, element=w518, error in (no error)=w522) -> (error out=w517:errorcluster)  [unwired: 1 in, 2 out]
            n233 = Merge Errors(w517, w515) -> (w516:errorcluster)
          }
          frame "Stop Motion" {
            n234 = Variant To Data(type=i16 0 ("GPIB Addresses.GPIB Motor"), Variant=w549) -> (data=w547:i16)  [unwired: 1 in, 1 out]
            n235 = call "ST - Stop motion.vi"("Axis"=i8 1, "Address / Port"=w547) -> ("error out"=w540:errorcluster, "Address / Port dup"=w539:i16)  [unwired: 7 in, 1 out]
            n236 = call "ST - Stop motion.vi"("error in"=w540, "Axis"=i8 2, "Address / Port"=w539) -> ("error out"=w538:errorcluster)  [unwired: 6 in, 2 out]
            n237 = To Variant(anything=-1) -> (Variant=w545:variant)
            n238 = Bundle("Consumer loop - States"=Consumer_loop_-_States."Idle", "Variant"=w545) -> (w543:T16)  [unwired: 1 in]
            n239 = Enqueue Element(queue=w550, element=w543, error in (no error)=w551) -> (error out=w542:errorcluster)  [unwired: 1 in, 2 out]
            n240 = Merge Errors(w542, w538) -> (w541:errorcluster)
          }
          frame "Disable buttons" {
            w558 = T7."Disabled and Grayed Out" ("Disabled")
            n241 = property on="Move" class="Bool"("DisabledEnum"=w558) -> ()  [unwired: 2 in, 2 out]
            n242 = property on="Right" class="Bool (strict)"("DisabledEnum"=w558) -> ()  [unwired: 2 in, 2 out]
            n243 = property on="Left" class="Bool (strict)"("DisabledEnum"=w558) -> ()  [unwired: 2 in, 2 out]
            n244 = property on="Up" class="Bool (strict)"("DisabledEnum"=w558) -> ()  [unwired: 2 in, 2 out]
            n245 = property on="Down" class="Bool (strict)"("DisabledEnum"=w558) -> ()  [unwired: 2 in, 2 out]
            n246 = Bundle("Consumer loop - States"=Consumer_loop_-_States."Check if move done", w553) -> (w556:cluster{"Consumer loop - States":T4, variant})  [unwired: 1 in]
            n247 = Enqueue Element(queue=w555, element=w556, error in (no error)=w554) -> (error out=w552:errorcluster)  [unwired: 1 in, 2 out]
          }
          frame "Check if move done" {
            n248 = Variant To Data(type=i16 0 ("Address / Port"), Variant=w575) -> (data=w561:i16)  [unwired: 1 in, 1 out]
            n249 = call "MD - Read motion done status.vi"("Axis"=i8 1, "Address / Port"=w561) -> ("Done"=w571:bool, "Address / Port dup"=w572:i16)  [unwired: 6 in, 2 out]
            n250 = call "MD - Read motion done status.vi"("Axis"=i8 2, "Address / Port"=w572) -> ("Done"=w570:bool)  [unwired: 6 in, 3 out]
            n251 = To Variant(anything=w561) -> (Variant=w560:variant)
            n252 = And(x=w570, y=w571) -> (x .and. y?=w567:bool)
            n253 = Select(t=Consumer_loop_-_States."Enable buttons" ("Consumer loop - States"), s=w567, f=Consumer_loop_-_States."Check if move done") -> (s? t:f=w564:T4)
            n254 = Bundle("f"=w564, "Variant"=w560) -> (w565:cluster{"f":T4, "Variant":variant})  [unwired: 1 in]
            n255 = Wait (ms)(milliseconds to wait=u32 100) -> ()  [unwired: 1 out]
            n256 = Enqueue Element(queue=w569, element=w565, error in (no error)=w568) -> (error out=w559:errorcluster)  [unwired: 1 in, 2 out]
          }
          frame "Enable buttons" {
            w579 = T7."Enabled" ("Disabled")
            n257 = property on="Move" class="Bool"("DisabledEnum"=w579) -> ()  [unwired: 2 in, 2 out]
            n258 = property on="Right" class="Bool (strict)"("DisabledEnum"=w579) -> ()  [unwired: 2 in, 2 out]
            n259 = property on="Left" class="Bool (strict)"("DisabledEnum"=w579) -> ()  [unwired: 2 in, 2 out]
            n260 = property on="Up" class="Bool (strict)"("DisabledEnum"=w579) -> ()  [unwired: 2 in, 2 out]
            n261 = property on="Down" class="Bool (strict)"("DisabledEnum"=w579) -> ()  [unwired: 2 in, 2 out]
            n262 = Bundle("Consumer loop - States"=Consumer_loop_-_States."Idle", w578) -> (w581:cluster{"Consumer loop - States":T4, variant})  [unwired: 1 in]
            n263 = Enqueue Element(queue=w583, element=w581, error in (no error)=w582) -> (error out=w577:errorcluster)  [unwired: 1 in, 2 out]
          }
          frame "Irradiation - Stop" {
            n264 = Variant To Data(type=T3 {"GPIB Addresses"={"GPIB Motor"=2, "GPIB Laser"="3"}, "Beam size"={"BeamX"=0.0, "BeamY"=0.0, "Beam Overlap"=0.0}, "Motor speed"={"Xspeed"=0.0, " Yspeed"=0.0}, "Laser parameters"={"Thyratron Bias"=20.0, "Frequency"=1, "Shots/Point"=1.0}, "Irradiation points"={"X1"=0.0, "Y1"=0.0, "X2"=0.0, "Y2"=0.0}, "Calibration Point"={"Xcalib"=0.0, "Ycalib"=0.0}} ("User Interface data"), Variant=w599) -> (data=w589:T3)  [unwired: 1 in, 1 out]
            n265 = Unbundle By Name(w589) -> ("GPIB Addresses.GPIB Motor"=w587:i16, "GPIB Addresses.GPIB Laser"=w588:string)
            n266 = Flush Queue(queue=w595, error in (no error)=w585) -> (queue out=w586:refnum<queue>, error out=w584:errorcluster)  [unwired: 1 out]
            n267 = call "Play laser.vi"("Laser On"=FALSE, "GPIB Address"=w588) -> ("Error Out"=w590:errorcluster)  [unwired: 8 in, 1 out]
            n268 = call "ST - Stop motion.vi"("error in"=w590, "Axis"=i8 1, "Address / Port"=w587) -> ("error out"=w605:errorcluster, "Address / Port dup"=w604:i16)  [unwired: 6 in, 1 out]
            n269 = To Variant(anything=-1) -> (Variant=w592:variant)
            n270 = call "ST - Stop motion.vi"("error in"=w605, "Axis"=i8 2, "Address / Port"=w604) -> ("error out"=w596:errorcluster)  [unwired: 6 in, 2 out]
            n271 = Bundle("Consumer loop - States"=Consumer_loop_-_States."Irradiation - Enable buttons", "Variant"=w592) -> (w594:T16)  [unwired: 1 in]
            n272 = Enqueue Element At Opposite End(queue=w586, element=w594, error in (no error)=w584) -> (error out=w597:errorcluster)  [unwired: 1 in, 2 out]
            n273 = Merge Errors(w597, w596) -> (w598:errorcluster)
          }
          frame "Irradiation - Check points" {
            n274 = Variant To Data(type=T3 {"GPIB Addresses"={"GPIB Motor"=2, "GPIB Laser"="3"}, "Beam size"={"BeamX"=0.0, "BeamY"=0.0, "Beam Overlap"=0.0}, "Motor speed"={"Xspeed"=0.0, " Yspeed"=0.0}, "Laser parameters"={"Thyratron Bias"=20.0, "Frequency"=1, "Shots/Point"=1.0}, "Irradiation points"={"X1"=0.0, "Y1"=0.0, "X2"=0.0, "Y2"=0.0}, "Calibration Point"={"Xcalib"=0.0, "Ycalib"=0.0}} ("User Interface data"), Variant=w625) -> (data=w619:T3)  [unwired: 1 in, 1 out]
            n275 = Unbundle By Name(w619) -> ("Irradiation points.X2"=w618:dbl, "Irradiation points.X1"=w617:dbl, "Irradiation points.Y2"=w615:dbl, "Irradiation points.Y1"=w616:dbl)
            n276 = Greater Or Equal?(x=w618, y=w617) -> (x >= y?=w614:bool)
            n277 = Less Or Equal?(x=w615, y=w616) -> (x <= y?=w613:bool)
            n278 = And(x=w614, y=w613) -> (x .and. y?=w607:bool)
            n279 = To Variant(anything=w619) -> (Variant=w620:variant)
            n280 = Not(x=w607) -> (.not. x?=w606:bool)
            n281 = Select(t=Consumer_loop_-_States."Irradiation - Disable buttons" ("Consumer loop - States"), s=w607, f=Consumer_loop_-_States."Idle") -> (s? t:f=w609:T4)
            n282 = Bundle("f"=w609, "Variant"=w620) -> (w623:cluster{"f":T4, "Variant":variant})  [unwired: 1 in]
            n283 = call "Display Message to User"("Enable"=w606, "Message"="Error!\nCheck the position of your points") -> ()  [unwired: 8 in, 2 out]
            n284 = Enqueue Element(queue=w622, element=w623, error in (no error)=w621) -> (error out=w612:errorcluster)  [unwired: 1 in, 2 out]
          }
          frame "Irradiation - Disable buttons" {
            w632 = T7."Disabled and Grayed Out" ("Disabled")
            n285 = property on="Move" class="Bool"("DisabledEnum"=w632) -> ()  [unwired: 2 in, 2 out]
            n286 = property on="Right" class="Bool (strict)"("DisabledEnum"=w632) -> ()  [unwired: 2 in, 2 out]
            n287 = property on="Left" class="Bool (strict)"("DisabledEnum"=w632) -> ()  [unwired: 2 in, 2 out]
            n288 = property on="Up" class="Bool (strict)"("DisabledEnum"=w632) -> ()  [unwired: 2 in, 2 out]
            n289 = property on="Down" class="Bool (strict)"("DisabledEnum"=w632) -> ()  [unwired: 2 in, 2 out]
            n290 = Bundle("Consumer loop - States"=Consumer_loop_-_States."Irradiation - Init position", w626) -> (w628:cluster{"Consumer loop - States":T4, variant})  [unwired: 1 in]
            n291 = Enqueue Element(queue=w631, element=w628, error in (no error)=w630) -> (error out=w629:errorcluster)  [unwired: 1 in, 2 out]
          }
          frame "Irradiation - Init position" {
            n292 = Variant To Data(type=T3 {"GPIB Addresses"={"GPIB Motor"=2, "GPIB Laser"="3"}, "Beam size"={"BeamX"=0.0, "BeamY"=0.0, "Beam Overlap"=0.0}, "Motor speed"={"Xspeed"=0.0, " Yspeed"=0.0}, "Laser parameters"={"Thyratron Bias"=20.0, "Frequency"=1, "Shots/Point"=1.0}, "Irradiation points"={"X1"=0.0, "Y1"=0.0, "X2"=0.0, "Y2"=0.0}, "Calibration Point"={"Xcalib"=0.0, "Ycalib"=0.0}} ("User Interface data"), Variant=w650) -> (data=w636:T3)  [unwired: 1 in, 1 out]
            n293 = Unbundle By Name(w636) -> ("GPIB Addresses.GPIB Laser"=w647:string, "GPIB Addresses.GPIB Motor"=w648:i16)
            n294 = Unbundle By Name(w636) -> ("Irradiation points.X1"=w646:dbl, "Irradiation points.Y1"=w645:dbl, "Laser parameters.Thyratron Bias"=w643:dbl, "Laser parameters.Frequency"=w644:u16)
            n295 = call "VA -Set velocity.vi"("Velocity\nset"=20.0 ("Velocity\nset"), "Axis #"=i8 1, "Address / Port"=w648) -> ("error out"=w655:errorcluster, "Address / Port dup"=w654:i16)  [unwired: 5 in, 2 out]
            n296 = Bundle("Thyratron Bias"=w643, "Frequency"=w644) -> (w642:cluster{"Thyratron Bias":dbl, "Frequency":u16})  [unwired: 1 in]
            n297 = To Variant(anything=w636) -> (Variant=w637:variant)
            n298 = call "VA -Set velocity.vi"("error in"=w655, "Velocity\nset"=20.0 ("Velocity\nset"), "Axis #"=i8 2, "Address / Port"=w654) -> ("error out"=w653:errorcluster, "Address / Port dup"=w652:i16)  [unwired: 4 in, 2 out]
            n299 = call "PA -Move to absolute position.vi"("Move to absolute\nposition - set"=w646, "error in"=w653, "Axis #"=i8 1, "Address / Port"=w652) -> ("error out"=w661:errorcluster, "Address / Port dup"=w660:i16)  [unwired: 2 in, 2 out]
            n300 = call "PA -Move to absolute position.vi"("Move to absolute\nposition - set"=w645, "error in"=w661, "Axis #"=i8 2, "Address / Port"=w660) -> ("error out"=w651:errorcluster)  [unwired: 2 in, 3 out]
            n301 = Bundle("Consumer loop - States"=Consumer_loop_-_States."Irradiation - Check if done", "Variant"=w637) -> (w639:T16)  [unwired: 1 in]
            n302 = call "Laser setup.vi"("Error In"=w651, "Laser Parameters"=w642, "GPIB Address"=w647) -> ("Error Out"=w635:errorcluster)  [unwired: 7 in, 1 out]
            n303 = Enqueue Element(queue=w641, element=w639, error in (no error)=w640) -> (error out=w634:errorcluster)  [unwired: 1 in, 2 out]
            n304 = Merge Errors(w634, w635) -> (w633:errorcluster)
          }
          frame "Irradiation - Check if done" {
            n305 = Variant To Data(type=T3 {"GPIB Addresses"={"GPIB Motor"=2, "GPIB Laser"="3"}, "Beam size"={"BeamX"=0.0, "BeamY"=0.0, "Beam Overlap"=0.0}, "Motor speed"={"Xspeed"=0.0, " Yspeed"=0.0}, "Laser parameters"={"Thyratron Bias"=20.0, "Frequency"=1, "Shots/Point"=1.0}, "Irradiation points"={"X1"=0.0, "Y1"=0.0, "X2"=0.0, "Y2"=0.0}, "Calibration Point"={"Xcalib"=0.0, "Ycalib"=0.0}} ("User Interface data"), Variant=w685) -> (data=w670:T3)  [unwired: 1 in, 1 out]
            n306 = Unbundle By Name(w670) -> ("GPIB Addresses.GPIB Motor"=w677:i16)
            n307 = call "MD - Read motion done status.vi"("Axis"=i8 1, "Address / Port"=w677) -> ("error out"=w678:errorcluster, "Done"=w673:bool, "Address / Port dup"=w681:i16)  [unwired: 6 in, 1 out]
            n308 = call "MD - Read motion done status.vi"("error in"=w678, "Axis"=i8 2, "Address / Port"=w681) -> ("error out"=w665:errorcluster, "Done"=w672:bool)  [unwired: 5 in, 2 out]
            n309 = To Variant(anything=w670) -> (Variant=w669:variant)
            n310 = And(x=w672, y=w673) -> (x .and. y?=w676:bool)
            n311 = Select(t=Consumer_loop_-_States."Irradiation - Sweep X", s=w676, f=Consumer_loop_-_States."Irradiation - Check if done" ("Consumer loop - States")) -> (s? t:f=w671:T4)
            n312 = Bundle("Consumer loop - States"=w671, "Variant"=w669) -> (w668:T16)  [unwired: 1 in]
            n313 = Wait (ms)(milliseconds to wait=u32 100) -> ()  [unwired: 1 out]
            n314 = Enqueue Element(queue=w683, element=w668, error in (no error)=w682) -> (error out=w666:errorcluster)  [unwired: 1 in, 2 out]
            n315 = Merge Errors(w666, w665) -> (w667:errorcluster)
          }
          frame "Irradiation - Sweep X" {
            n316 = Variant To Data(type=T3 {"GPIB Addresses"={"GPIB Motor"=2, "GPIB Laser"="3"}, "Beam size"={"BeamX"=0.0, "BeamY"=0.0, "Beam Overlap"=0.0}, "Motor speed"={"Xspeed"=0.0, " Yspeed"=0.0}, "Laser parameters"={"Thyratron Bias"=20.0, "Frequency"=1, "Shots/Point"=1.0}, "Irradiation points"={"X1"=0.0, "Y1"=0.0, "X2"=0.0, "Y2"=0.0}, "Calibration Point"={"Xcalib"=0.0, "Ycalib"=0.0}} ("User Interface data"), Variant=w701) -> (data=w689:T3)  [unwired: 1 in, 1 out]
            n317 = Unbundle By Name(w689) -> ("GPIB Addresses.GPIB Motor"=w695:i16, "GPIB Addresses.GPIB Laser"=w696:string)
            n318 = Unbundle By Name(w689) -> ("Motor speed.Xspeed"=w688:dbl, "Irradiation points.X2"=w687:dbl, "Irradiation points.X1"=w686:dbl)
            n319 = call "Play laser.vi"("Laser On"=TRUE, "GPIB Address"=w696) -> ("Error Out"=w708:errorcluster)  [unwired: 8 in, 1 out]
            n320 = To Variant(anything=w689) -> (Variant=w697:variant)
            n321 = call "VA -Set velocity.vi"("error in"=w708, "Velocity\nset"=w688, "Axis #"=i8 1, "Address / Port"=w695) -> ("error out"=w704:errorcluster, "Axis # dup"=w705:i8, "Address / Port dup"=w706:i16)  [unwired: 4 in, 1 out]
            n322 = Subtract(x=w687, y=w686) -> (x-y=w707:dbl)
            n323 = call "PR - Move to relative position.vi"("error in"=w704, "Nstep"=w707, "Axis  #"=w705, "Address / Port"=w706) -> ("error out"=w690:errorcluster)  [unwired: 3 in, 2 out]
            n324 = Bundle("Consumer loop - States"=Consumer_loop_-_States."Irradiation - Check X", "Variant"=w697) -> (w693:T16)  [unwired: 1 in]
            n325 = Enqueue Element(queue=w699, element=w693, error in (no error)=w698) -> (error out=w692:errorcluster)  [unwired: 1 in, 2 out]
            n326 = Merge Errors(w692, w690) -> (w691:errorcluster)
          }
          frame "Irradiation - Check X" {
            n327 = Variant To Data(type=T3 {"GPIB Addresses"={"GPIB Motor"=2, "GPIB Laser"="3"}, "Beam size"={"BeamX"=0.0, "BeamY"=0.0, "Beam Overlap"=0.0}, "Motor speed"={"Xspeed"=0.0, " Yspeed"=0.0}, "Laser parameters"={"Thyratron Bias"=20.0, "Frequency"=1, "Shots/Point"=1.0}, "Irradiation points"={"X1"=0.0, "Y1"=0.0, "X2"=0.0, "Y2"=0.0}, "Calibration Point"={"Xcalib"=0.0, "Ycalib"=0.0}} ("User Interface data"), Variant=w724) -> (data=w715:T3)  [unwired: 1 in, 1 out]
            n328 = Unbundle By Name(w715) -> ("GPIB Addresses.GPIB Motor"=w723:i16)
            n329 = call "MD - Read motion done status.vi"("Axis"=i8 1, "Address / Port"=w723) -> ("error out"=w709:errorcluster, "Done"=w719:bool)  [unwired: 6 in, 2 out]
            n330 = To Variant(anything=w715) -> (Variant=w714:variant)
            n331 = Select(t=Consumer_loop_-_States."Irradiation - Check Y" ("Consumer loop - States"), s=w719, f=Consumer_loop_-_States."Irradiation - Check X") -> (s? t:f=w712:T4)
            n332 = Bundle("f"=w712, "Variant"=w714) -> (w713:cluster{"f":T4, "Variant":variant})  [unwired: 1 in]
            n333 = Enqueue Element(queue=w716, element=w713, error in (no error)=w717) -> (error out=w711:errorcluster)  [unwired: 1 in, 2 out]
            n334 = Wait (ms)(milliseconds to wait=u32 100) -> ()  [unwired: 1 out]
            n335 = Merge Errors(w711, w709) -> (w710:errorcluster)
          }
          frame "Irradiation - Check Y" {
            # "#debugged? Testare un po'"
            n336 = Variant To Data(type=T3 {"GPIB Addresses"={"GPIB Motor"=2, "GPIB Laser"="3"}, "Beam size"={"BeamX"=0.0, "BeamY"=0.0, "Beam Overlap"=0.0}, "Motor speed"={"Xspeed"=0.0, " Yspeed"=0.0}, "Laser parameters"={"Thyratron Bias"=20.0, "Frequency"=1, "Shots/Point"=1.0}, "Irradiation points"={"X1"=0.0, "Y1"=0.0, "X2"=0.0, "Y2"=0.0}, "Calibration Point"={"Xcalib"=0.0, "Ycalib"=0.0}} ("User Interface data"), Variant=w748) -> (data=w741:T3)  [unwired: 1 in, 1 out]
            n337 = Unbundle By Name(w741) -> ("GPIB Addresses.GPIB Motor"=w729:i16, "GPIB Addresses.GPIB Laser"=w747:string)
            n338 = Unbundle By Name(w741) -> ("Beam size.BeamY"=w733:dbl, "Beam size.Beam Overlap"=w734:dbl, "Irradiation points.Y2"=w735:dbl)
            n339 = call "Play laser.vi"("Laser On"=FALSE, "GPIB Address"=w747) -> ("Error Out"=w730:errorcluster)  [unwired: 8 in, 1 out]
            n340 = call "TP - Read actual position.vi"("error in"=w730, "Axis"=i8 2, "Address / Port"=w729) -> ("error out"=w726:errorcluster, "Query the current actual\nposition - read"=w727:dbl)  [unwired: 5 in, 2 out]
            n341 = Subtract(x=w733, y=w734) -> (x-y=w732:dbl)
            n342 = To Variant(anything=w741) -> (Variant=w740:variant)
            n343 = Subtract(x=w727, y=w732) -> (x-y=w731:dbl)
            n344 = Greater Or Equal?(x=w731, y=w735) -> (x >= y?=w746:bool)
            n345 = Select(t=Consumer_loop_-_States."Irradiation - Sweep Y" ("Consumer loop - States"), s=w746, f=Consumer_loop_-_States."Irradiation - Enable buttons") -> (s? t:f=w738:T4)
            n346 = Bundle("f"=w738, "Variant"=w740) -> (w739:cluster{"f":T4, "Variant":variant})  [unwired: 1 in]
            n347 = Enqueue Element(queue=w742, element=w739, error in (no error)=w743) -> (error out=w737:errorcluster)  [unwired: 1 in, 2 out]
            n348 = Merge Errors(w737, w726) -> (w736:errorcluster)
          }
          frame "Irradiation - Sweep Y" {
            n349 = Variant To Data(type=T3 {"GPIB Addresses"={"GPIB Motor"=2, "GPIB Laser"="3"}, "Beam size"={"BeamX"=0.0, "BeamY"=0.0, "Beam Overlap"=0.0}, "Motor speed"={"Xspeed"=0.0, " Yspeed"=0.0}, "Laser parameters"={"Thyratron Bias"=20.0, "Frequency"=1, "Shots/Point"=1.0}, "Irradiation points"={"X1"=0.0, "Y1"=0.0, "X2"=0.0, "Y2"=0.0}, "Calibration Point"={"Xcalib"=0.0, "Ycalib"=0.0}} ("User Interface data"), Variant=w774) -> (data=w765:T3)  [unwired: 1 in, 1 out]
            n350 = Unbundle By Name(w765) -> ("Beam size.BeamY"=w763:dbl, "Beam size.Beam Overlap"=w764:dbl, "Irradiation points.X1"=w755:dbl)
            n351 = Unbundle By Name(w765) -> ("GPIB Addresses.GPIB Motor"=w766:i16)
            n352 = Subtract(x=w763, y=w764) -> (x-y=w752:dbl)
            n353 = Negate(x=w752) -> (-x=w751:dbl)
            n354 = To Variant(anything=w765) -> (Variant=w768:variant)
            n355 = call "PR - Move to relative position.vi"("Nstep"=w751, "Axis  #"=i8 2, "Address / Port"=w766) -> ("error out"=w760:errorcluster, "Address / Port dup"=w759:i16)  [unwired: 4 in, 1 out]
            n356 = call "VA -Set velocity.vi"("error in"=w760, "Velocity\nset"=20.0 ("Velocity\nset"), "Axis #"=i8 1, "Address / Port"=w759) -> ("error out"=w756:errorcluster, "Address / Port dup"=w757:i16)  [unwired: 4 in, 2 out]
            n357 = Bundle("Consumer loop - States"=Consumer_loop_-_States."Irradiation - Check if done", "Variant"=w768) -> (w769:T16)  [unwired: 1 in]
            n358 = call "PA -Move to absolute position.vi"("Move to absolute\nposition - set"=w755, "error in"=w756, "Axis #"=i8 1, "Address / Port"=w757) -> ("error out"=w754:errorcluster)  [unwired: 2 in, 3 out]
            n359 = Enqueue Element(queue=w773, element=w769, error in (no error)=w772) -> (error out=w771:errorcluster)  [unwired: 1 in, 2 out]
            n360 = Merge Errors(w771, w754) -> (w770:errorcluster)
          }
          frame "Irradiation - Enable buttons" {
            w784 = T7."Enabled" ("Disabled")
            n361 = property on="Move" class="Bool"("DisabledEnum"=w784) -> ()  [unwired: 2 in, 2 out]
            n362 = property on="Right" class="Bool (strict)"("DisabledEnum"=w784) -> ()  [unwired: 2 in, 2 out]
            n363 = property on="Left" class="Bool (strict)"("DisabledEnum"=w784) -> ()  [unwired: 2 in, 2 out]
            n364 = To Variant(anything=w777) -> (Variant=w781:variant)
            n365 = property on="Up" class="Bool (strict)"("DisabledEnum"=w784) -> ()  [unwired: 2 in, 2 out]
            n366 = property on="Down" class="Bool (strict)"("DisabledEnum"=w784) -> ()  [unwired: 2 in, 2 out]
            n367 = local write "Irradiate"(FALSE ("Irradiate")) -> ()
            n368 = Bundle("Consumer loop - States"=Consumer_loop_-_States."Idle", "Variant"=w781) -> (w783:T16)  [unwired: 1 in]
            n369 = Enqueue Element(queue=w779, element=w783, error in (no error)=w780) -> (error out=w778:errorcluster)  [unwired: 1 in, 2 out]
          }
        }
        n370 = Unbundle By Name(w404) -> ("status"=w403:bool)
        n371 = call "All close.vi"("Close? (F)"=w403) -> ("Close"=w405:bool)  [unwired: 9 in, 1 out]
      }
      frame Error {
        n372 = Unbundle By Name(w791) -> ("GPIB Addresses.GPIB Motor"=w787:i16, "GPIB Addresses.GPIB Laser"=w786:string)
        n373 = call "AB - Abort Motion.vi"("error in"=w788, "Address / Port"=w787) -> ("error out"=w790:errorcluster)  [unwired: 9 in]
        n374 = call "Play laser.vi"("Error In"=w790, "Laser On"=FALSE, "GPIB Address"=w786) -> ("Error Out"=w785:errorcluster)  [unwired: 7 in, 1 out]
      }
    }
  }
  n375 = while {
    tunnel: w10 -> [w800]
    tunnel: w7 -> [w799]
    tunnel: [w798] -> w6
    tunnel: [w796] -> w5
    stop <- w793 stop-if-true
    n376 = event shown="[1] \"Motor Enable\": Value Change" {
      selector: _ -> [_ _ _]
      dyn-events: _ -> [_ _ _]
      timeout: 500 -> [_ _ _]
      tunnel: w800 -> [w803 w810 w813]
      tunnel: w799 -> [w802 w809 w812]
      tunnel: [w803 w808 w813] -> w798
      tunnel: [w802 w807 w812] -> w796
      tunnel: [FALSE FALSE TRUE] -> w795
      event Timeout {
        n377 = event-data() -> ()  [unwired: 1 in, 1 out]
      }
      event "Motor Enable": Value Change {
        n378 = event-data() -> ("NewVal"=w805:bool)  [unwired: 1 in]
        n379 = call-poly <vilib>:"Digital Write.vi"("Error In"=w809, "Output Value"=w805, "DO Channel"=u8 7, "LINX Resource"=w810) -> ("Error Out"=w807:errorcluster, "LINX Resource"=w808:T8)  [unwired: 6 in]
      }
      event "Exit": Value Change; Panel Close {
        n380 = event-data() -> ()  [unwired: 1 in, 1 out]
      }
    }
    n381 = Or(x=w796, y=w795) -> (x .or. y?=w794:bool)
    n382 = call "All close.vi"("Close? (F)"=w794) -> ("Close"=w793:bool)  [unwired: 9 in, 1 out]
  }
  n383 = call-poly <vilib>:"Digital Write.vi"("Error In"=w5, "Output Value"=FALSE, "DO Channel"=u8 7, "LINX Resource"=w6) -> ("Error Out"=w3:errorcluster, "LINX Resource"=w4:T8)  [unwired: 6 in]
  n384 = call <vilib>:"IMAQdx Close Camera.vi"("error in"=w34, "Session In"=w35) -> ()  [unwired: 9 in, 1 out]
  n385 = Release Queue(queue=w21, error in (no error)=w22) -> ()  [unwired: 1 in, 3 out]
  n386 = call <vilib>:"Close.vi"("Error In"=w3, "LINX Resource"=w4) -> ()  [unwired: 9 in, 1 out]
